vi "Interfaz grafica - corriente.vi"() -> ()   [LabVIEW 2024]
uses:
  160620 Optotune Lens Driver 4 Labview package/Hello Optotune Lens (30.06.2015)/Calibration.ctl
  <vilib>/DAQmx/read.llb/DAQmx Read (Analog 1D Wfm NChan NSamp).vi
  <vilib>/Analysis/2dsp.llb/Decimate (single shot, DBL).vi
  <vilib>/Utility/file.llb/Read Delimited Spreadsheet (string).vi
  <vilib>/Instr/_visa.llb/VISA Configure Serial Port (Instr).vi
  <vilib>/DAQmx/create/channels.llb/DAQmx Create Channel (AI-Voltage-Basic).vi
  <vilib>/DAQmx/configure/timing.llb/DAQmx Timing (Sample Clock).vi
  <vilib>/DAQmx/miscellaneous.llb/DAQmx Fill In Error Info.vi
  <vilib>/Waveform/WDTOps.llb/WDT Index Channel DBL.vi
  <vilib>/Analysis/2dsp.llb/Decimate (continuous, DBL).vi
  <vilib>/Utility/file.llb/Write Delimited Spreadsheet (string).vi
  <vilib>/Waveform/WDTOps.llb/WDT Get Waveform Time Array DBL.vi
  <vilib>/Analysis/NI_AALPro.lvlib
panel:
  out "Array 4":string[](array[string])
  out "Array 3":string[](array[string])
  out "Array 2":string[](array[string])
  out "Array":string[](array[string])
  out "Nombre 2":string
  in  "Restablecer Iniciales":bool
  in  "Incremento":dbl=0.1 format="%#_13g"
  out "Potencia derecho":dbl
  out "error out 4":errorcluster
  out "error out 3":errorcluster
  out "error out 2":errorcluster
  in  "Tab Control 3":enum32{"WL", "Video"}(tab)
  out "Waveform length":dbl[][](graph)
  in  "Minimo escala Y":dbl format="%#_13g"
  in  "Maximo escala Y":dbl format="%#_13g"
  in  "Escala autom. Y":u8=1
  in  "Escala autom. X":u8=1
  in  "Maximo escala X":dbl
  in  "Minimo escala X":dbl
  out "VISA resource name out":string
  in  "Tab Control 2":T1(tab)
  in  "DAQmx Physical Channel":tag
  in  "Frecuencia muestreo":i32=20000
  in  "tamaño buffer":i32=1000
  in  "factor decimacion":i32=20
  in  "Ganancia":u16(ring) items=["0.2"=51455, "1"=33023, "10"=49407, "20"=41215, "30"=57599, "40"=37119, "60"=53503, "80"=45311, "120"=61695, "157"=35071, ""=0]
  in  "Potencia inicial lente derecho":dbl(slide) scale=-3.0..3.0
  in  "Potencia inicial lente izquierdo":dbl(slide) scale=-3.0..3.0
  in  "VISA resource name":string="COM11"
  in  "VISA resource name 2":string="COM10"
  out "DPT INICIALES D":dbl
  out "DPT INICIALES I":dbl
  out "Potencia izquierdo":dbl
  in  "error in (no error) 5":errorcluster
  in  "error in (no error) 4":errorcluster
  in  "error in (no error) 3":errorcluster
  in  "error in (no error) 2":errorcluster
  in  "Calibration 4":T2={"Max Current A"=293.0, "Max Current B"=293.0, "UCL A"=300.0, "UCL B"=300.0, "LCL A"=0.0, "LCL B"=0.0} {"Max Current A" format="%#_g mA"; "Max Current B" format="%#_g mA"; "UCL A" format="%#_g mA"; "LCL A" format="%#_g mA"; "UCL B" format="%#_g mA"; "LCL B" format="%#_g mA"}
  out "ID 2":u16
  out "VISA resource name out 2":string
  out "Calibration 3":T2 {"Max Current A" format="%#_g mA"; "Max Current B" format="%#_g mA"; "UCL A" format="%#_g mA"; "LCL A" format="%#_g mA"; "UCL B" format="%#_g mA"; "LCL B" format="%#_g mA"}
  out "OK 2":bool
  out "Data 2":string
  out "Command to Port 2":string
  in  "Cola tipo 2":dbl[](array[numeric])
  out "Distancia":u32
  in  "Tamaño ventana WL":i32=60
  in  "Limite inferior WL":dbl=25.0 format="%#_13g"
  in  "Limite superior WL":dbl=50.0
  out "number":u32
  in  "Calibration":T2={"Max Current A"=293.0, "Max Current B"=293.0, "UCL A"=300.0, "UCL B"=300.0, "LCL A"=0.0, "LCL B"=0.0} {"Max Current A" format="%#_g mA"; "Max Current B" format="%#_g mA"; "UCL A" format="%#_g mA"; "LCL A" format="%#_g mA"; "UCL B" format="%#_g mA"; "LCL B" format="%#_g mA"}
  out "ID":u16
  out "Calibration 2":T2 {"Max Current A" format="%#_g mA"; "Max Current B" format="%#_g mA"; "UCL A" format="%#_g mA"; "LCL A" format="%#_g mA"; "UCL B" format="%#_g mA"; "LCL B" format="%#_g mA"}
  out "OK":bool
  out "Data":string
  out "Command to Port":string
  in  "DPT dif.":dbl
  out "error out":errorcluster
  in  "error in (no error)":errorcluster
  in  "WL":dbl
  in  "Cola tipo":dbl[](array[numeric])
  out "T button?":bool
  in  "Elegir menu Exp":bool
  in  "Elegir menu":bool
  out "path":path
  in  "Iniciar experimento":bool
  in  "Parar adquisicion":bool
  out "Enfermedad visual":string
  out "Edad":string
  out "Nombre":string
  out "Cedula":string
  in  "Carpeta":path=path "C:/Users/TGM1603/Documents/LabVIEW Data/Experimentos electrodos"
  in  "?":bool
  in  "Menu Principal":u16(ring) items=["Visualizacion general ", "Llevar a cabo un experimento", "Ajustar potencia inicial lentes"]
  in  "Menu experimentos":u16(ring) items=["Experimento 1", "Experimento 2", "Experimento 3", "Experimento 4"]
  in  "Tab Control":enum32{"Señal EMG", "Potencia y distancia"}(tab)
  out "Senal EMG":waveform(dbl)[](graph)
  in  "Escala automatica Y":u8
  in  "Escala automatica X":u8=1
  in  "X Scale.Range:Increment":dbl
  in  "X Scale.Range:Minimum":dbl
  in  "X Scale.Range:Maximum":dbl
  in  "Y Scale.Range:Minimum":dbl=-5.0
  in  "Y Scale.Range:Maximum":dbl=5.0
  in  "Escala Y min":dbl
  in  "Escala Y max":dbl
  in  "Auto scale Y":u8=1
  in  "Escala X max":dbl
  in  "Escala X min":dbl
  out "Potencia optica y distancia":dbl[][](graph)
  in  "Auto scale X":u8=1
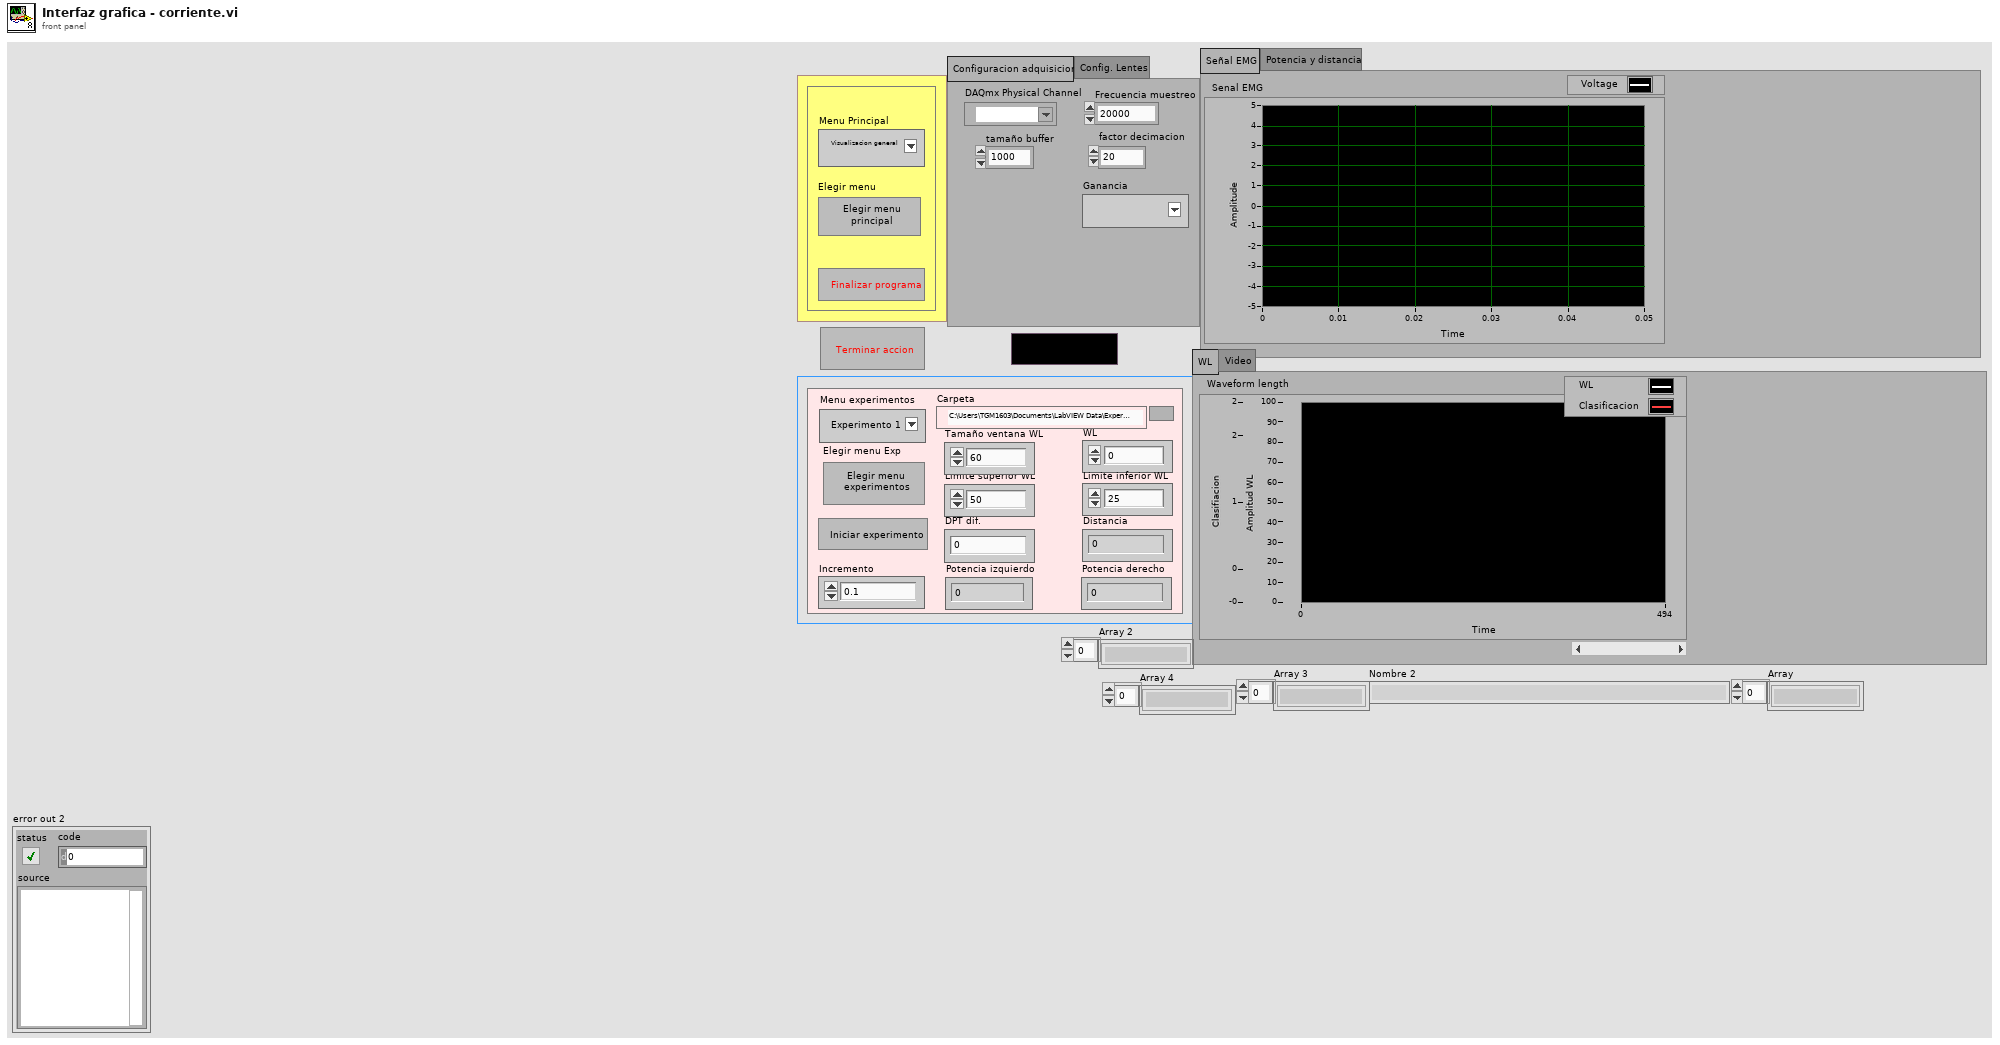
[diagram p1: front panel]
types:
  T1 = enum32{"Configuracion adquisicion", "Config. Lentes"}
  T2 = typedef "Calibration.ctl" = cluster{"Max Current A":dbl, "Max Current B":dbl, "UCL A":dbl, "UCL B":dbl, "LCL A":dbl, "LCL B":dbl}
  T3 = enum16{"Left Button", "Center Button", "Right Button", "Window Close"}
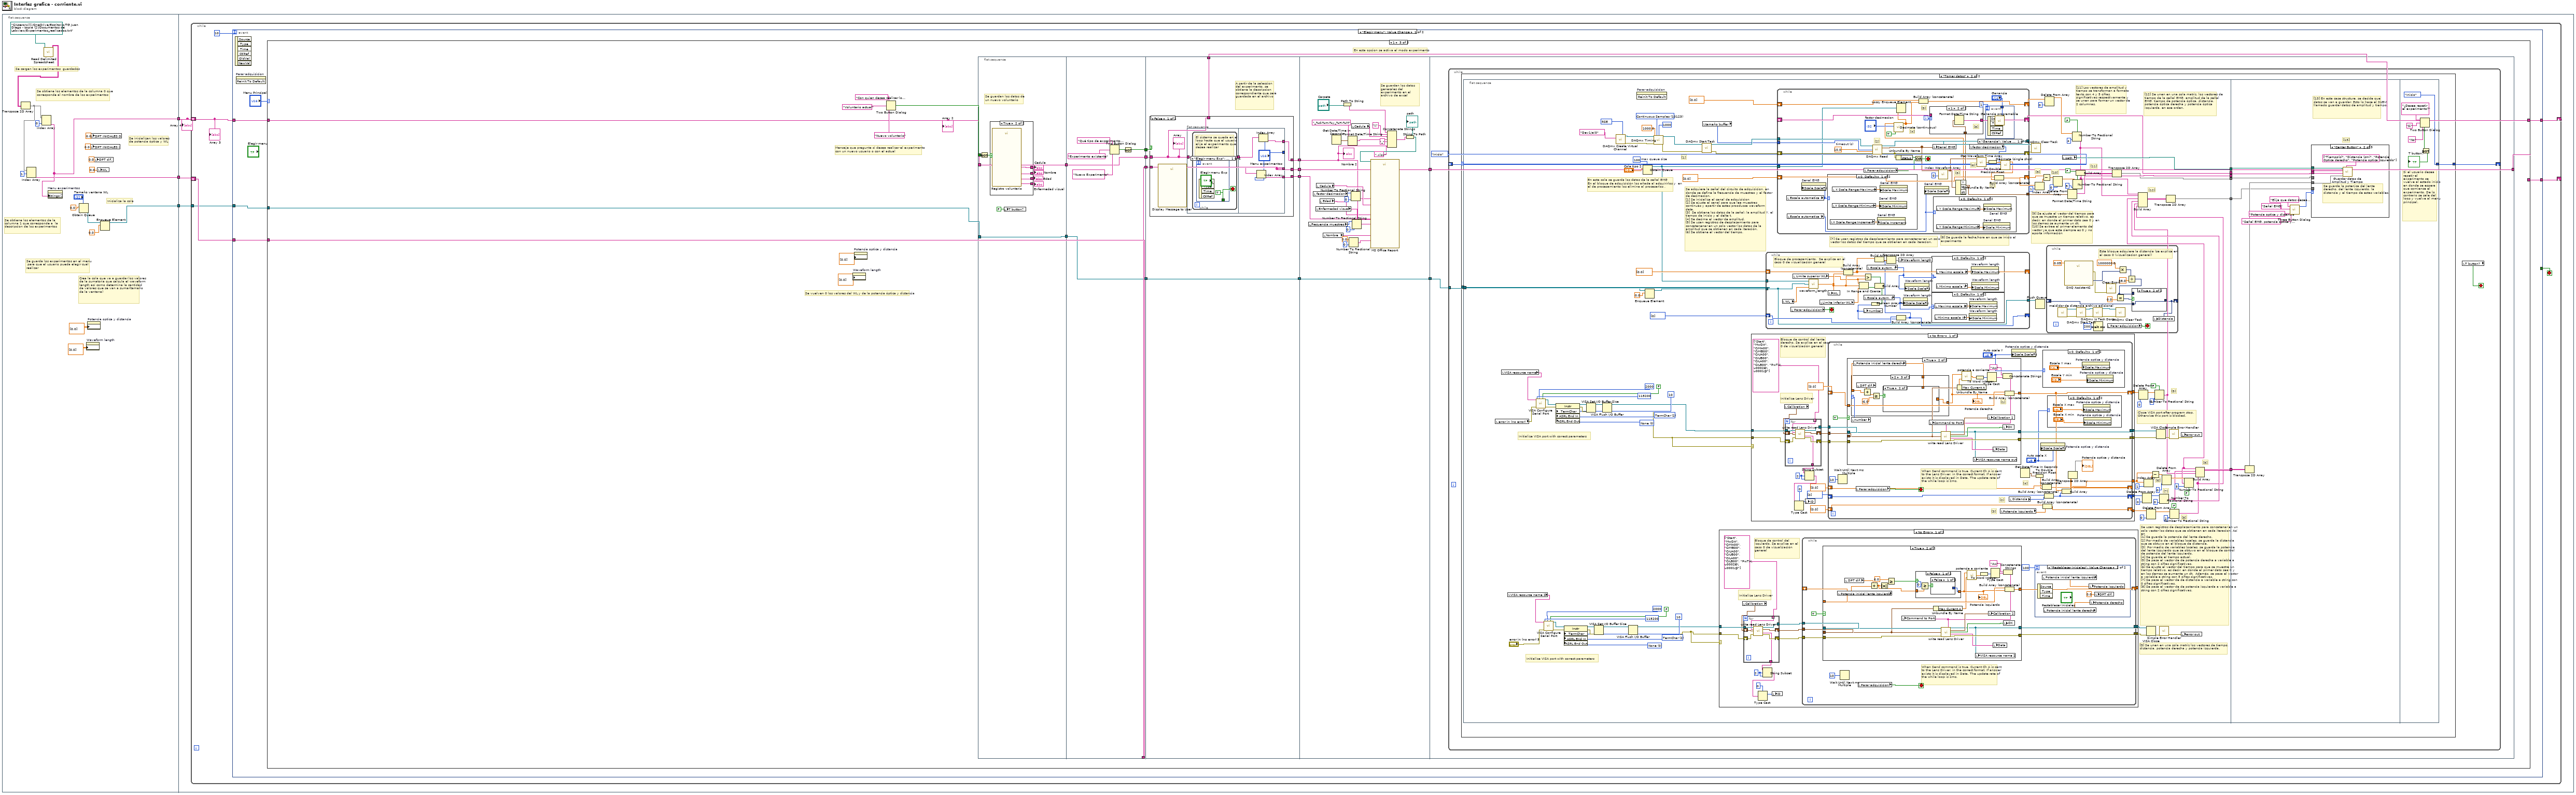
[diagram p0: block diagram]
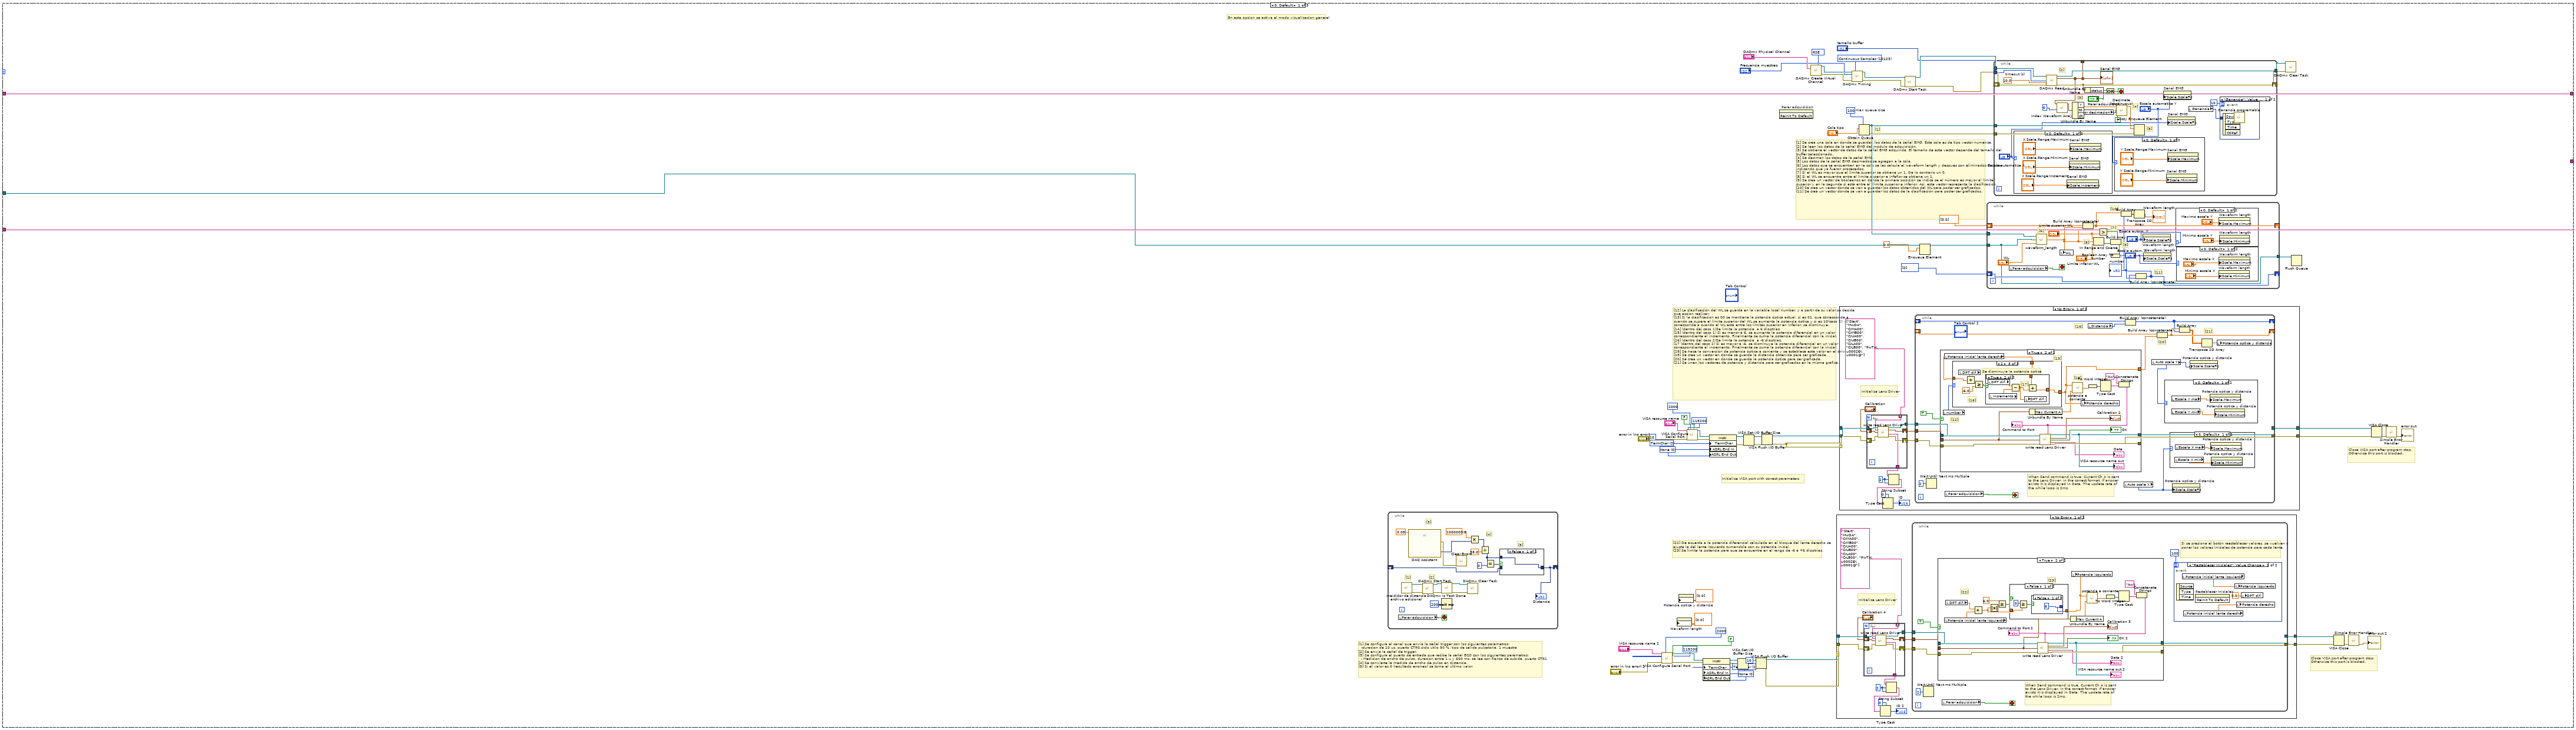
[diagram p2: hidden frame]
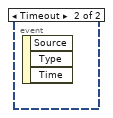
[diagram p3: hidden frame]
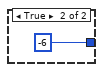
[diagram p5: hidden frame]
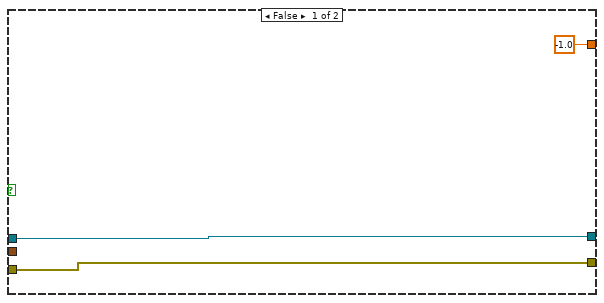
[diagram p11: hidden frame]
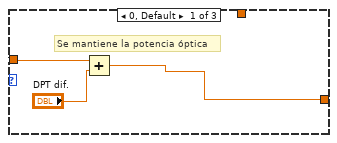
[diagram p12: hidden frame]
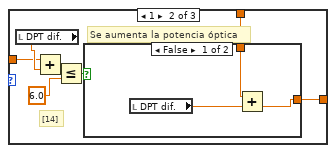
[diagram p13: hidden frame]
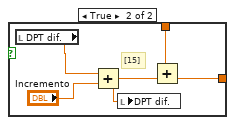
[diagram p14: hidden frame]
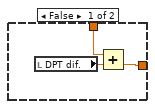
[diagram p15: hidden frame]
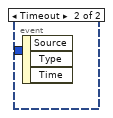
[diagram p19: hidden frame]
diagram:
  n1 = flat-sequence {
    tunnel: [w18] -> w3
    tunnel: [w15] -> w2
    tunnel: [w10] -> w1
    tunnel: w3 -> [w22]
    tunnel: w2 -> [w24]
    tunnel: w1 -> [w23]
    frame #0 {
      # "Se inicializan los valores\nde potencia óptica y WL"
      # "Inicializa la cola"
      # "Crea la cola que va a guardar los valores de la sumatoria que calcula el waveform length así como determina la cantidad de valores que se van a sumar(tamaño de la ventana)"
      # "Se obtiene los elementos de la columna 1 que corresponde a  la descripcion de los experimentos"
      # "Se obtiene los elementos de la columna 0 que corresponde al nombre de los experimentos"
      # "Se guarda los experimentos en el menu\n para que el usuario pueda elegir cual \nrealizar"
      # "Se cargan los experimentos  guardados"
      n2 = call-poly <vilib>:"Read Delimited Spreadsheet.vi"("file path (dialog if empty)"=path "C:/Users/willi/OneDrive/Escritorio/TG Juan Diego - copia (2)/Documentos de Labview/Experimentos_realizados.txt") -> ("all rows"=w19:string[][])  [unwired: 9 in, 5 out]
      n3 = Transpose 2D Array(2D array=w19) -> (transposed array=w16:string[][])
      n4 = Index Array(array=w16, index (row)=1) -> (element=w15:string[])  [unwired: 1 in]
      n5 = Index Array(array=w16, index (row)=0) -> (element=w18:string[])  [unwired: 1 in]
      n6 = property on="Menu experimentos" class="Ring (strict)"("Strings []"=w18) -> ()  [unwired: 2 in, 2 out]
      n7 = Obtain Queue(max queue size (-1, unlimited)="Tamaño ventana WL", element data type=0.0) -> (queue out=w13:refnum<queue>)  [unwired: 3 in, 2 out]
      n8 = property on="Waveform length" class="WFChart (strict)"("History Data"=dbl[][] [[0.0]]) -> ()  [unwired: 2 in, 2 out]
      n9 = property on="Potencia optica y distancia" class="WFChart (strict)"("History Data"=dbl[][] [[0.0]]) -> ()  [unwired: 2 in, 2 out]
      n10 = local write "DPT INICIALES D"(0.0 ("DPT INIT.1")) -> ()
      n11 = local write "DPT INICIALES I"(0.0 ("DPT INIT.2")) -> ()
      n12 = local write "DPT dif."(0.0 ("WL")) -> ()
      n13 = local write "WL"(0.0 ("WL")) -> ()
      n14 = Enqueue Element(queue=w13, element=0.0) -> (queue out=w10:refnum<queue>)  [unwired: 2 in, 2 out]
    }
    frame #1 {
      n15 = while {
        shift-right: [w30] -> _
        shift-left: w22 -> [w31]
        shift-right: [w28] -> _
        shift-left: w24 -> [w29]
        tunnel: w23 -> [w27]
        stop <- w26 stop-if-true
        n16 = event shown="[0] \"Elegir menu\": Value Change" {
          selector: _ -> [_ _]
          dyn-events: _ -> [_ _]
          timeout: 10 -> [_ _]
          tunnel: w31 -> [w37 w1042]
          tunnel: [w36 w1042] -> w30
          tunnel: w29 -> [w35 w1041]
          tunnel: [w34 w1041] -> w28
          tunnel: w27 -> [w32 _]
          tunnel: [_ "?"] -> w26
          event "Elegir menu": Value Change {
            n17 = event-data() -> ()  [unwired: 1 in, 6 out]
            n18 = invoke on="Parar adquisicion" class="Bool (strict)" method="Reinit To Default"() -> ()  [unwired: 3 in, 3 out]
            n19 = case shown="1" "Menu Principal" {
              tunnel: w37 -> [w104 w383 w503]
              tunnel: [w104 w383 w502] -> w36
              tunnel: w35 -> [w103 w382 w500]
              tunnel: [w103 w382 w499] -> w34
              tunnel: w32 -> [w93 _ w490]
              frame 0, Default {
                w38 = 10123 items=["Finite Samples"=10178, "Continuous Samples"=10123, "Hardware Timed Single Point"=12522] ("sample mode")
                w39 = 10083 items=["Default"=-1, "RSE"=10083, "NRSE"=10078, "Differential"=10106, "Pseudodifferential"=12529] ("input terminal configuration")
                w61 = u16 0 items=["None", "Last Bit", "TermChar", "Break"] ("Serial Settings:End Mode for Writes")
                w60 = u16 2 items=["None", "Last Bit", "TermChar"] ("Serial Settings:End Mode for Reads")
                w83 = u16 0 items=["None", "Last Bit", "TermChar", "Break"] ("Serial Settings:End Mode for Writes")
                w84 = u16 2 items=["None", "Last Bit", "TermChar"] ("Serial Settings:End Mode for Reads")
                w97 = 100  # max queue size
                # "[22] De acuerda a la potencia diferencial calculada en el bloque del lente derecho se ajusta la del lente izquierdo sumandola con su potencia inicial.\n[23] Se limita la potencia para que se encuentre en el rango de -6 a +6 dioptrías."
                # "[12] La clasificación del WL se guarda en la variable local number, y a partir de su valor se decide que accion realizar.\n[13] Si la clasificacion es 00 se mantiene la potencia óptica actual, si es 01, que corresponde a cuando se supera el limite superior del WL,se aumenta la potencia óptica y si es 10(caso 2), que corresponde a cuando el WL está entre los limites superior en inferior, se disminuye. \n[14] (dentro del caso 1)Se limita la potencia  a 6 dioptrías. \n[15] (dentro del caso 1) Si es menor a 6, se aumenta la potencia diferencial en un valor correspondiente al incremento. Finalmente se suma la potencia diferencial con la inicial.\n[16] (dentro del caso 2)Se limita la potencia  a -6 dioptrías.\n[17 (dentro del caso 2) Si es mayor a -6, se disminuye la potencia diferencial en un valor correspondiente al incremento. Finalmente se suma la potencia diferencial con la inicial.\n[18] Se hace la conversión de potencia óptica a corriente y se establece este valor en el driver.\n[19] Se crea un vector en donde se guarda la distancia obtenida para ser graficada.\n[20] Se crea un vector en donde se guarda la potencia óptica para ser graficada.\n[21] Se unen los vectores de potencia y distancia para ser graficados en la misma grafica."
                # "[1] Se crea una cola en donde se guardan los datos de la señal EMG. Esta cola es de tipo vector numerica.\n[2] Se leen los datos de la señal EMG del módulo de adquisición. \n[3] Se obtiene el vector de datos de la señal EMG adquirida. El tamaño de este vector depende del tamaño del buffer seleccionado.\n[4] Se deciman los datos de la señal EMG.\n[5] Los datos de la señal EMG decimados se agregan a la cola.\n[6] Los datos que se encuentran en la cola se les calcula el waveform length y después son eliminados de esta, indicando que ya fueron procesados. \n[7] Si el WL es mayor que el limite superior se obtiene un 1. De lo contrario un 0.\n[8] Si el WL se encuentra entre el límite superior e infefior se obtiene un 1.\n[9] Se crea un vector de booleanos en donde la primera posición se indica se el número es mayor al límite superior y en la segunda si está entre el  limite superior e inferior. Así, este vector representa la clasificación.\n[10] Se crea un vector donde se van a guardar los datos obtenidos del WL para poder ser graficados.\n[11] Se crea un vector donde se van a guardar los datos de la clasificación para poder ser graficados."
                # "[1]"
                # "En esta opcion se activa el modo visualizacion general"
                # "Close VISA port after program stop. Otherwise this port is blocked."
                # "[1] Se configura el canal que envía la señal trigger con los siguientes parametros:\n  -duracion de 10 us, puerto CTR0,ciclo utilo 50 %, tipo de salida pulsatoria, 1 muestra \n[2] Se envía la señal de trigger.\n[3] Se configura el puerto de entrada que recibe la señal ECO con los siguientes parámetros:\n  - Medicion de ancho de pulso, duracion entre 1 u y 600 ms, se lee con flanco de subida, puerto CTR1\n[4] Se convierte la medida de ancho de pulso en distancia.\n[5] Si el valor es 0 (resultado erroneo) se toma el último valor."
                # "Close VISA port after program stop. Otherwise this port is blocked."
                # "Initialize VISA port with correct parameters"
                n20 = while {
                  shift-right: [w172] -> _
                  shift-left: _ -> [w171]
                  stop <- w176 stop-if-true
                  # "[5]"
                  # "[4]"
                  # "[3]"
                  # "[2]"
                  # "[1]"
                  n21 = local read "Parar adquisicion"() -> (w176:bool)
                  n22 = call "meididor de distancia archivo adicional.vi"() -> ("error out"=w179:errorcluster, "task out"=w180:refnum<k21>)  [unwired: 10 in]
                  n23 = call "DAQ Assistant"("timeout (s)"=0.05) -> ("data"=w189:dynamicdata, "error out"=w177:errorcluster)  [unwired: 16 in, 1 out]
                  n24 = call <vilib>:"DAQmx Start Task.vi"("task/channels in"=w180, "error in"=w179) -> ("task out"=w183:refnum<k21>, "error out"=w184:errorcluster)  [unwired: 12 in]
                  n25 = call <vilib>:"DAQmx Is Task Done.vi"("task/channels in"=w183, "error in"=w184) -> ("task out"=w181:refnum<k21>, "error out"=w182:errorcluster)  [unwired: 11 in, 1 out]
                  n26 = Wait (ms)(milliseconds to wait=u32 200) -> ()  [unwired: 1 out]
                  n27 = call <vilib>:"Clear Errors.vi"("error in (no error)"=w177) -> ()  [unwired: 5 in, 2 out]
                  n28 = call <vilib>:"DAQmx Clear Task.vi"("task in"=w181, "error in"=w182) -> ()  [unwired: 13 in, 1 out]
                  n29 = Multiply(x=1000000.0, y=w189) -> (x*y=w187:dynamicdata)
                  n30 = Divide(x=w187, y=58.0) -> (x/y=w173:dynamicdata)
                  n31 = Equal?(x=w173, y=u16 0) -> (x = y?=w175:dynamicdata)
                  n32 = case shown="False" w175 {
                    tunnel: [w190 w191] -> w172
                    tunnel: w173 -> [w190 _]
                    tunnel: w171 -> [_ w191]
                    frame False {
                    }
                    frame True {
                    }
                  }
                  "Distancia" <- w172
                }
                n33 = call-poly "VISA Configure Serial Port"("VISA resource name"="VISA resource name 2", "timeout (10sec)"=u32 2000, "Enable Termination\nChar (T)"=FALSE ("Enable Termination\nChar (T)"), "baud rate (9600)"=u32 115200, "error in (no error)"="error in (no error) 2") -> ("VISA resource name out"=w56:refnum<visa-resource-name>, "error out"=w58:errorcluster)  [unwired: 9 in]
                n34 = property on="Waveform length" class="WFChart (strict)"("History Data"=dbl[][] [[0.0]]) -> ()  [unwired: 2 in, 2 out]
                n35 = property on="Potencia optica y distancia" class="WFChart (strict)"("History Data"=dbl[][] [[0.0]]) -> ()  [unwired: 2 in, 2 out]
                n36 = call-poly "VISA Configure Serial Port"("VISA resource name"="VISA resource name", "timeout (10sec)"=u32 2000, "Enable Termination\nChar (T)"=FALSE ("Enable Termination\nChar (T)"), "baud rate (9600)"=u32 115200, "error in (no error)"="error in (no error)") -> ("VISA resource name out"=w88:refnum<visa-resource-name>, "error out"=w86:errorcluster)  [unwired: 9 in]
                n37 = property class="Instr"(reference=w56, error in=w58, "TermChar"=u8 10 ("Message Based Settings:Termination Character"), "ASRL End In"=w60, "ASRL End Out"=w61) -> (reference out=w57:refnum<visa-resource-name>, error out=w59:errorcluster)
                n38 = property class="Instr"(reference=w88, error in=w86, "TermChar"=u8 10 ("Message Based Settings:Termination Character"), "ASRL End In"=w84, "ASRL End Out"=w83) -> (reference out=w87:refnum<visa-resource-name>, error out=w85:errorcluster)
                n39 = VISA Set I/O Buffer Size(VISA resource name=w57, error in (no error)=w59) -> (VISA resource name out=w64:refnum<visa-resource-name>, error out=w65:errorcluster)  [unwired: 2 in]
                n40 = VISA Set I/O Buffer Size(VISA resource name=w87, error in (no error)=w85) -> (VISA resource name out=w80:refnum<visa-resource-name>, error out=w79:errorcluster)  [unwired: 2 in]
                n41 = VISA Flush I/O Buffer(VISA resource name=w64, error in (no error)=w65) -> (VISA resource name out=w50:refnum<visa-resource-name>, error out=w51:errorcluster)  [unwired: 1 in]
                n42 = VISA Flush I/O Buffer(VISA resource name=w80, error in (no error)=w79) -> (VISA resource name out=w78:refnum<visa-resource-name>, error out=w73:errorcluster)  [unwired: 1 in]
                n43 = invoke on="Parar adquisicion" class="Bool (strict)" method="Reinit To Default"() -> ()  [unwired: 3 in, 3 out]
                n44 = call-poly <vilib>:"DAQmx Create Virtual Channel.vi"("input terminal configuration"=w39, "physical channels"="DAQmx Physical Channel") -> ("task out"=w45:refnum<k21>, "error out"=w44:errorcluster)  [unwired: 12 in]
                n45 = case shown="No Error" w51 {
                  tunnel: w51 -> [w118 w169]
                  tunnel: w50 -> [w117 w170]
                  tunnel: [w116 w169] -> w46
                  tunnel: [w115 w170] -> w47
                  frame No Error {
                    w113 = 2 ("length (rest)")
                    # "Initialize Lens Driver"
                    n46 = for {
                      tunnel: w117 -> [w167]
                      tunnel: [w164] -> w107
                      tunnel: string[] ["Start", "MwDA", "CrMA00", "CrMB00", "CrUA00", "CrUB00", "CrLA00", "CrLB00", "PwTA\u0002Ð\u0001@"] -> [w162] mode=indexing
                      tunnel: [w161] -> w106
                      shift-right: [w165] -> w108
                      shift-left: "Calibration 4" -> [w166]
                      shift-right: [w163] -> w109
                      shift-left: w118 -> [w168]
                      n47 = call "write read Lens Driver.vi"("VISA resource name"=w167, "command"=w162, "Calibration"=w166, "error in (no error)"=w168) -> ("VISA resource name out"=w164:refnum<visa-resource-name>, "Calibration 2"=w165:T2, "Data"=w161:string, "error out"=w163:errorcluster)  [unwired: 4 in, 4 out]
                    }
                    n48 = String Subset(string=w106, offset (0)=w113, length (rest)=w113) -> (substring=w111:string)
                    n49 = Type Cast(type=u16 0 ("length (rest)"), x=w111) -> (*(type *) &x=→"ID 2":u16)
                    n50 = while {
                      tunnel: [w121] -> w116
                      tunnel: [w122] -> w115
                      tunnel: w109 -> [w127]
                      tunnel: w108 -> [w126]
                      tunnel: w107 -> [w125]
                      stop <- w120 stop-if-true
                      # "Si se presiona el botón reestablecer valores, se vuelven a poner los valores iniciales de potencia para cada lente"
                      # "When Send command is true, Current Ch A is sent to the Lens Driver, in the correct format. If answer exists it is displayed in Data. The update rate of the while loop is 2ms."
                      n51 = Wait Until Next ms Multiple(millisecond multiple=u32 2) -> ()  [unwired: 1 out]
                      n52 = case shown="True" TRUE ("Send command") {
                        tunnel: [w132 w153] -> w121
                        tunnel: w127 -> [w132 w152]
                        tunnel: w126 -> [_ w134]
                        tunnel: w125 -> [w131 w151]
                        tunnel: [w131 w148] -> w122
                        frame False {
                        }
                        frame True {
                          # "[23]"
                          # "[22]"
                          n53 = local read "Potencia inicial lente izquierdo"() -> (w142:dbl)
                          n54 = local read "DPT dif."() -> (w143:dbl)
                          n55 = Add(x=w143, y=w142) -> (x+y=w138:dbl)
                          n56 = Absolute Value(x=w138) -> (abs(x)=w140:dbl)
                          n57 = Greater Or Equal?(x=6.0, y=w140) -> (x >= y?=w141:bool)
                          n58 = case shown="False" w141 {
                            tunnel: w138 -> [w156 w160]
                            tunnel: [w154 w160] -> w136
                            frame False {
                              n59 = Greater Or Equal?(x=u16 0, y=w156) -> (x >= y?=w157:bool)
                              n60 = case shown="False" w157 {
                                tunnel: [i16 6 ("x") i16 -6 ("x")] -> w154
                                frame False {
                                }
                                frame True {
                                }
                              }
                            }
                            frame True {
                            }
                          }
                          n61 = Unbundle By Name(w134) -> ("Max Current A"=w135:dbl)
                          n62 = local write "Potencia izquierdo"(w136) -> ()
                          n63 = call "potencia a corriente.vi"("Max current A"=w135, "Potencia"=w136) -> ("Corriente"=w137:dbl)
                          n64 = To Word Integer(number=w137) -> (16bit integer=w146:i16)
                          n65 = Type Cast(x=w146) -> (*(type *) &x=w145:string)  [unwired: 1 in]
                          n66 = Concatenate Strings("Aw", w145) -> (w144:string)
                          "Command to Port 2" <- w144
                          n67 = call "write read Lens Driver.vi"("VISA resource name"=w151, "command"=w144, "Calibration"=w134, "error in (no error)"=w152) -> ("VISA resource name out"=w148:refnum<visa-resource-name>, "Calibration 2"=→"Calibration 3":T2, "OK"=→"OK 2":bool, "Data"=→"Data 2":string, "error out"=w153:errorcluster)  [unwired: 4 in, 3 out]
                          "VISA resource name out 2" <- w148
                        }
                      }
                      n68 = local read "Parar adquisicion"() -> (w120:bool)
                      n69 = event shown="[0] \"Restablecer Iniciales\": Value Change" {
                        selector: _ -> [_ _]
                        dyn-events: _ -> [_ _]
                        timeout: 100 -> [_ _]
                        event "Restablecer Iniciales": Value Change {
                          n70 = event-data() -> ()  [unwired: 1 in, 3 out]
                          n71 = local read "Potencia inicial lente izquierdo"() -> (w128:dbl)
                          n72 = local read "Potencia inicial lente derecho"() -> (w129:dbl)
                          n73 = invoke on="Restablecer Iniciales" class="Bool" method="Reinit To Default"() -> ()  [unwired: 3 in, 3 out]
                          n74 = local write "Potencia izquierdo"(w128) -> ()
                          n75 = local write "Potencia derecho"(w129) -> ()
                          n76 = local write "DPT dif."(0.0 ("DPT dif.")) -> ()
                        }
                        event Timeout {
                          n77 = event-data() -> ()  [unwired: 1 in, 3 out]
                        }
                      }
                    }
                  }
                  frame Error {
                  }
                }
                n78 = case shown="No Error" w73 {
                  tunnel: w73 -> [w205 w289]
                  tunnel: w78 -> [w204 w290]
                  tunnel: [w203 w289] -> w76
                  tunnel: [w202 w290] -> w74
                  frame No Error {
                    w200 = 2 ("length (rest)")
                    # "Initialize Lens Driver"
                    n79 = for {
                      tunnel: w204 -> [w287]
                      tunnel: [w284] -> w194
                      tunnel: string[] ["Start", "MwDA", "CrMA00", "CrMB00", "CrUA00", "CrUB00", "CrLA00", "CrLB00", "PwTA\u0002Ð\u0001@"] -> [w282] mode=indexing
                      tunnel: [w281] -> w193
                      shift-right: [w285] -> w195
                      shift-left: "Calibration" -> [w286]
                      shift-right: [w283] -> w196
                      shift-left: w205 -> [w288]
                      n80 = call "write read Lens Driver.vi"("VISA resource name"=w287, "command"=w282, "Calibration"=w286, "error in (no error)"=w288) -> ("VISA resource name out"=w284:refnum<visa-resource-name>, "Calibration 2"=w285:T2, "Data"=w281:string, "error out"=w283:errorcluster)  [unwired: 4 in, 4 out]
                    }
                    n81 = String Subset(string=w193, offset (0)=w200, length (rest)=w200) -> (substring=w198:string)
                    n82 = Type Cast(type=u16 0 ("length (rest)"), x=w198) -> (*(type *) &x=→"ID":u16)
                    n83 = while {
                      tunnel: [w217] -> w203
                      tunnel: [w218] -> w202
                      tunnel: w196 -> [w223]
                      tunnel: w195 -> [w222]
                      tunnel: w194 -> [w221]
                      shift-right: [w208] -> _
                      shift-left: _ -> [w212]
                      shift-right: [w209] -> _
                      shift-left: _ -> [w211]
                      stop <- w216 stop-if-true
                      # "[21]"
                      # "[20]"
                      # "[19]"
                      # "When Send command is true, Current Ch A is sent to the Lens Driver, in the correct format. If answer exists it is displayed in Data. The update rate of the while loop is 2ms."
                      n84 = Wait Until Next ms Multiple(millisecond multiple=u32 2) -> ()  [unwired: 1 out]
                      n85 = case shown="True" TRUE ("Send command") {
                        tunnel: [w230 w247] -> w217
                        tunnel: w223 -> [w230 w246]
                        tunnel: w222 -> [_ w233]
                        tunnel: w221 -> [w229 w245]
                        tunnel: [w229 w242] -> w218
                        tunnel: [-1.0 ("DPT") w235] -> w210
                        frame False {
                        }
                        frame True {
                          # "[18]"
                          # "[13]"
                          # "[12]"
                          n86 = local read "number"() -> (w237:u32)
                          n87 = local read "Potencia inicial lente derecho"() -> (w236:dbl)
                          n88 = case shown="2" w237 {
                            tunnel: [w249 w257 w272] -> w235
                            tunnel: w236 -> [w250 w252 w267]
                            tunnel: w236 -> [_ w251 w266]
                            frame 0, Default {
                              # "Se mantiene la potencia óptica"
                              n89 = Add(x=w250, y="DPT dif.") -> (x+y=w249:dbl)
                            }
                            frame 1 {
                              # "[14]"
                              # "Se aumenta la potencia óptica"
                              n90 = local read "DPT dif."() -> (w253:dbl)
                              n91 = Add(x=w252, y=w253) -> (x+y=w254:dbl)
                              n92 = Less Or Equal?(x=w254, y=6.0) -> (x <= y?=w256:bool)
                              n93 = case shown="False" w256 {
                                tunnel: [w259 w262] -> w257
                                tunnel: w251 -> [w258 w261]
                                frame False {
                                n94 = local read "DPT dif."() -> (w260:dbl)
                                n95 = Add(x=w258, y=w260) -> (x+y=w259:dbl)
                                }
                                frame True {
                                # "[15]"
                                n96 = local read "DPT dif."() -> (w263:dbl)
                                n97 = Add(x=w263, y="Incremento") -> (x+y=w264:dbl)
                                n98 = local write "DPT dif."(w264) -> ()
                                n99 = Add(x=w261, y=w264) -> (x+y=w262:dbl)
                                }
                              }
                            }
                            frame 2 {
                              # "[16]"
                              # "Se disminuye la potencia óptica"
                              n100 = local read "DPT dif."() -> (w271:dbl)
                              n101 = Add(x=w271, y=w267) -> (x+y=w268:dbl)
                              n102 = Greater Or Equal?(x=w268, y=-6.0) -> (x >= y?=w269:bool)
                              n103 = case shown="True" w269 {
                                tunnel: [w274 w278] -> w272
                                tunnel: w266 -> [w273 w277]
                                frame False {
                                n104 = local read "DPT dif."() -> (w275:dbl)
                                n105 = Add(x=w273, y=w275) -> (x+y=w274:dbl)
                                }
                                frame True {
                                # "[17]"
                                n106 = local read "DPT dif."() -> (w280:dbl)
                                n107 = local read "Incremento"() -> (w276:dbl)
                                n108 = Subtract(x=w280, y=w276) -> (x-y=w279:dbl)
                                n109 = local write "DPT dif."(w279) -> ()
                                n110 = Add(x=w277, y=w279) -> (x+y=w278:dbl)
                                }
                              }
                            }
                          }
                          n111 = Unbundle By Name(w233) -> ("Max Current A"=w232:dbl)
                          n112 = call "potencia a corriente.vi"("Max current A"=w232, "Potencia"=w235) -> ("Corriente"=w234:dbl)
                          n113 = local write "Potencia derecho"(w235) -> ()
                          n114 = To Word Integer(number=w234) -> (16bit integer=w240:i16)
                          n115 = Type Cast(x=w240) -> (*(type *) &x=w239:string)  [unwired: 1 in]
                          n116 = Concatenate Strings("Aw", w239) -> (w238:string)
                          "Command to Port" <- w238
                          n117 = call "write read Lens Driver.vi"("VISA resource name"=w245, "command"=w238, "Calibration"=w233, "error in (no error)"=w246) -> ("VISA resource name out"=w242:refnum<visa-resource-name>, "Calibration 2"=→"Calibration 2":T2, "OK"=→"OK":bool, "Data"=→"Data":string, "error out"=w247:errorcluster)  [unwired: 4 in, 3 out]
                          "VISA resource name out" <- w242
                        }
                      }
                      n118 = local read "Parar adquisicion"() -> (w216:bool)
                      n119 = local read "Distancia"() -> (w213:u32)
                      n120 = local read "Auto scale X"() -> (w214:u8)
                      n121 = Build Array (concatenate)(w212, w213) -> (w208:u32[])
                      n122 = local read "Auto scale Y"() -> (w215:u8)
                      n123 = Build Array (concatenate)(w211, w210) -> (w209:dbl[])
                      n124 = case shown="0, Default" w215 {
                        frame 0, Default {
                          n125 = local read "Escala Y max"() -> (w227:dbl)
                          n126 = local read "Escala Y min"() -> (w226:dbl)
                          n127 = property on="Potencia optica y distancia" class="WFChart (strict)"("YScale.Maximum"=w227) -> ()  [unwired: 2 in, 2 out]
                          n128 = property on="Potencia optica y distancia" class="WFChart (strict)"("YScale.Minimum"=w226) -> ()  [unwired: 2 in, 2 out]
                        }
                        frame 1 {
                        }
                      }
                      n129 = case shown="0, Default" w214 {
                        frame 0, Default {
                          n130 = local read "Escala X min"() -> (w224:dbl)
                          n131 = local read "Escala X max"() -> (w225:dbl)
                          n132 = property on="Potencia optica y distancia" class="WFChart (strict)"("XScale.Maximum"=w225) -> ()  [unwired: 2 in, 2 out]
                          n133 = property on="Potencia optica y distancia" class="WFChart (strict)"("XScale.Minimum"=w224) -> ()  [unwired: 2 in, 2 out]
                        }
                        frame 1 {
                        }
                      }
                      n134 = property on="Potencia optica y distancia" class="WFChart (strict)"("XScale.ScaleFit"=w214) -> ()  [unwired: 2 in, 2 out]
                      n135 = Build Array(w209, w208) -> (w207:dbl[][])
                      n136 = property on="Potencia optica y distancia" class="WFChart (strict)"("YScale.ScaleFit"=w215) -> ()  [unwired: 2 in, 2 out]
                      n137 = Transpose 2D Array(2D array=w207) -> (transposed array=w206:dbl[][])
                      n138 = local write "Potencia optica y distancia"(w206) -> ()
                    }
                  }
                  frame Error {
                  }
                }
                n139 = call-poly <vilib>:"DAQmx Timing.vi"("task/channels in"=w45, "sample mode"=w38, "rate"="Frecuencia muestreo", "error in"=w44) -> ("task out"=w43:refnum<k21>, "error out"=w42:errorcluster)  [unwired: 10 in]
                n140 = Obtain Queue(max queue size (-1, unlimited)=w97, element data type="Cola tipo") -> (queue out=w94:refnum<queue>, error out=w95:errorcluster)  [unwired: 3 in, 1 out]
                n141 = call <vilib>:"DAQmx Start Task.vi"("task/channels in"=w43, "error in"=w42) -> ("task out"=w102:refnum<k21>, "error out"=w101:errorcluster)  [unwired: 12 in]
                n142 = Enqueue Element(queue=w93, element=0.0) -> (queue out=w70:refnum<queue>)  [unwired: 2 in, 2 out]
                n143 = while {
                  tunnel: w70 -> [w292]
                  tunnel: w94 -> [w309]
                  shift-right: [w295] -> _
                  shift-left: dbl[] [0.0] -> [w306]
                  shift-right: [w294] -> _
                  shift-left: u32[] [0] -> [w296]
                  tunnel: [w292] -> w68
                  stop <- w307 stop-if-true
                  # "[11]"
                  # "[10]"
                  # "[9]"
                  # "[8]"
                  # "[7]"
                  # "[6]"
                  n144 = local read "Parar adquisicion"() -> (w307:bool)
                  n145 = call "waveform_length.vi"("WL"="WL", "Cola WL"=w292, "Datos entrada"=w309) -> ("WL 2"=w304:dbl)
                  n146 = local write "WL"(w304) -> ()
                  n147 = Build Array (concatenate)(w306, w304) -> (w295:dbl[])
                  n148 = In Range and Coerce(upper limit="Limite superior WL", x=w304, lower limit="Limite inferior WL") -> (In Range?=w302:bool)  [unwired: 1 out]
                  n149 = Greater?(x=w304, y="Limite superior WL") -> (0:w303:bool)
                  n150 = Build Array(w303, w302) -> (w301:bool[])
                  n151 = Boolean Array To Number(Boolean array=w301) -> (number=w297:u32)
                  "number" <- w297
                  n152 = Build Array (concatenate)(w296, w297) -> (w294:u32[])
                  n153 = Build Array(w295, w294) -> (w293:dbl[][])
                  n154 = Transpose 2D Array(2D array=w293) -> (transposed array=→"Waveform length":dbl[][])
                  n155 = property on="Waveform length" class="WFChart (strict)"("YScale.ScaleFit"="Escala autom. Y") -> ()  [unwired: 2 in, 2 out]
                  n156 = property on="Waveform length" class="WFChart (strict)"("XScale.ScaleFit"="Escala autom. X") -> ()  [unwired: 2 in, 2 out]
                  n157 = case shown="0, Default" "Escala autom. Y" {
                    frame 0, Default {
                      n158 = property on="Waveform length" class="WFChart (strict)"("YScale.Maximum"="Maximo escala Y") -> ()  [unwired: 2 in, 2 out]
                      n159 = property on="Waveform length" class="WFChart (strict)"("YScale.Minimum"="Minimo escala Y") -> ()  [unwired: 2 in, 2 out]
                    }
                    frame 1 {
                    }
                  }
                  n160 = case shown="0, Default" "Escala autom. X" {
                    frame 0, Default {
                      n161 = property on="Waveform length" class="WFChart (strict)"("XScale.Minimum"="Minimo escala X") -> ()  [unwired: 2 in, 2 out]
                      n162 = property on="Waveform length" class="WFChart (strict)"("XScale.Maximum"="Maximo escala X") -> ()  [unwired: 2 in, 2 out]
                    }
                    frame 1 {
                    }
                  }
                }
                n163 = while {
                  tunnel: w102 -> [w335]
                  tunnel: "tamaño buffer" -> [w332]
                  tunnel: [w333] -> w98
                  shift-right: [w330] -> w99
                  shift-left: w101 -> [w334]
                  tunnel: [w324] -> _
                  tunnel: w94 -> [w320]
                  tunnel: w95 -> [w319]
                  stop <- w329 stop-if-true
                  w328 = 10.0  # timeout (s)
                  # "[5]"
                  # "[4]"
                  # "[3]"
                  # "[2]"
                  n164 = case shown="0, Default" "Escala automatica X" {
                    frame 0, Default {
                      n165 = property on="Senal EMG" class="WFGraph (strict)"("XScale.Increment"="X Scale.Range:Increment") -> ()  [unwired: 2 in, 2 out]
                      n166 = property on="Senal EMG" class="WFGraph (strict)"("XScale.Minimum"="X Scale.Range:Minimum") -> ()  [unwired: 2 in, 2 out]
                      n167 = property on="Senal EMG" class="WFGraph (strict)"("XScale.Maximum"="X Scale.Range:Maximum") -> ()  [unwired: 2 in, 2 out]
                    }
                    frame 1 {
                    }
                  }
                  n168 = call-poly <vilib>:"DAQmx Read.vi"("task/channels in"=w335, "number of samples per channel"=w332, "timeout"=w328, "error in"=w334) -> ("task out"=w333:refnum<k21>, "data"=w324:waveform(dbl)[], "error out"=w330:errorcluster)  [unwired: 9 in]
                  "Senal EMG" <- w324
                  n169 = call-poly <vilib>:"Index Waveform Array.vi"("index"=0, "waveform array"=w324) -> ("waveform"=w325:waveform(dbl))  [unwired: 8 in, 1 out]
                  n170 = Unbundle By Name(w325) -> ("Y"=w322:dbl[])  [unwired: 2 out]
                  n171 = local read "factor decimacion"() -> (w321:i32)
                  n172 = Unbundle By Name(w330) -> ("status"=w331:bool)
                  n173 = Or(x=w331, y="Parar adquisicion") -> (x .or. y?=w329:bool)
                  n174 = case shown="0, Default" "Escala automatica Y" {
                    frame 0, Default {
                      n175 = property on="Senal EMG" class="WFGraph (strict)"("YScale.Minimum"="Y Scale.Range:Minimum") -> ()  [unwired: 2 in, 2 out]
                      n176 = property on="Senal EMG" class="WFGraph (strict)"("YScale.Maximum"="Y Scale.Range:Maximum") -> ()  [unwired: 2 in, 2 out]
                    }
                    frame 1 {
                    }
                  }
                  n177 = call-poly <vilib>:"Decimate (continuous).vi"("averaging"=TRUE, "decimating factor"=w321, "X"=w322) -> ("Decimated Array"=w318:dbl[])  [unwired: 7 in, 1 out]
                  n178 = Lossy Enqueue Element(queue=w320, element=w318, error in (no error)=w319) -> ()  [unwired: 4 out]
                  n179 = property on="Senal EMG" class="WFGraph (strict)"("YScale.ScaleFit"="Escala automatica Y") -> ()  [unwired: 2 in, 2 out]
                  n180 = property on="Senal EMG" class="WFGraph (strict)"("XScale.ScaleFit"="Escala automatica X") -> ()  [unwired: 2 in, 2 out]
                  n181 = local read "Ganancia"() -> (w315:u16)
                  n182 = event shown="[0] \"Ganancia\": Value Change" {
                    selector: _ -> [_ _]
                    dyn-events: _ -> [_ _]
                    timeout: 10 -> [_ _]
                    tunnel: w315 -> [w336 _]
                    event "Ganancia": Value Change {
                      n183 = event-data() -> ()  [unwired: 1 in, 4 out]
                      n184 = call "Ganancia programable.vi"("MOSI data"=w336) -> ()
                    }
                    event Timeout {
                      n185 = event-data() -> ()  [unwired: 1 in, 3 out]
                    }
                  }
                }
                n186 = call <vilib>:"DAQmx Clear Task.vi"("task in"=w98, "error in"=w99) -> ()  [unwired: 13 in, 1 out]
                n187 = Flush Queue(queue=w68) -> ()  [unwired: 1 in, 3 out]
                n188 = VISA Close(VISA resource name=w47, error in (no error)=w46) -> (error out=w48:errorcluster)
                n189 = call <vilib>:"Simple Error Handler.vi"("error in (no error)"=w48) -> ("error out"=→"error out 2":errorcluster)  [unwired: 4 in, 4 out]
                n190 = VISA Close(VISA resource name=w74, error in (no error)=w76) -> (error out=w77:errorcluster)
                n191 = call <vilib>:"Simple Error Handler.vi"("error in (no error)"=w77) -> ("error out"=→"error out":errorcluster)  [unwired: 4 in, 4 out]
              }
              frame 2 {
                w362 = u16 0 items=["None", "Last Bit", "TermChar", "Break"] ("Serial Settings:End Mode for Writes")
                w361 = u16 2 items=["None", "Last Bit", "TermChar"] ("Serial Settings:End Mode for Reads")
                w375 = u16 0 items=["None", "Last Bit", "TermChar", "Break"] ("Serial Settings:End Mode for Writes")
                w374 = u16 2 items=["None", "Last Bit", "TermChar"] ("Serial Settings:End Mode for Reads")
                # "En esta opcion se configura la potencia inicial de los lentes"
                # "Close VISA port after program stop. Otherwise this port is blocked."
                # "Close VISA port after program stop. Otherwise this port is blocked."
                # "PwTA command to set temperature limits: PwTA as ASCII characters followed by 45 and 20 degrees in binary code."
                # "Initialize VISA port with correct parameters"
                # "PwTA command to set temperature limits: PwTA as ASCII characters followed by 45 and 20 degrees in binary code."
                # "Initialize VISA port with correct parameters"
                n192 = local read "VISA resource name"() -> (w352:string)
                n193 = call-poly "VISA Configure Serial Port"("VISA resource name"=w352, "timeout (10sec)"=u32 2000, "Enable Termination\nChar (T)"=FALSE ("Enable Termination\nChar (T)"), "baud rate (9600)"=u32 115200, "error in (no error)"="error in (no error) 3") -> ("VISA resource name out"=w357:refnum<visa-resource-name>, "error out"=w359:errorcluster)  [unwired: 9 in]
                n194 = property class="Instr"(reference=w357, error in=w359, "TermChar"=u8 10 ("Message Based Settings:Termination Character"), "ASRL End In"=w361, "ASRL End Out"=w362) -> (reference out=w358:refnum<visa-resource-name>, error out=w360:errorcluster)
                n195 = VISA Set I/O Buffer Size(VISA resource name=w358, error in (no error)=w360) -> (VISA resource name out=w364:refnum<visa-resource-name>, error out=w365:errorcluster)  [unwired: 2 in]
                n196 = VISA Flush I/O Buffer(VISA resource name=w364, error in (no error)=w365) -> (VISA resource name out=w351:refnum<visa-resource-name>, error out=w350:errorcluster)  [unwired: 1 in]
                n197 = case shown="No Error" w350 {
                  tunnel: w350 -> [w397 w431]
                  tunnel: w351 -> [w396 w432]
                  tunnel: [w395 w431] -> w346
                  tunnel: [w394 w432] -> w347
                  frame No Error {
                    w393 = 2 ("length (rest)")
                    # "Initialize Lens Driver"
                    n198 = local read "Calibration"() -> (w385:T2)
                    n199 = for {
                      tunnel: w396 -> [w429]
                      tunnel: [w426] -> w388
                      tunnel: string[] ["Start", "MwDA", "CrMA00", "CrMB00", "CrUA00", "CrUB00", "CrLA00", "CrLB00", "PwTA\u0002Ð\u0001@"] -> [w424] mode=indexing
                      tunnel: [w423] -> w387
                      shift-right: [w427] -> w389
                      shift-left: w385 -> [w428]
                      shift-right: [w425] -> w390
                      shift-left: w397 -> [w430]
                      n200 = call "write read Lens Driver.vi"("VISA resource name"=w429, "command"=w424, "Calibration"=w428, "error in (no error)"=w430) -> ("VISA resource name out"=w426:refnum<visa-resource-name>, "Calibration 2"=w427:T2, "Data"=w423:string, "error out"=w425:errorcluster)  [unwired: 4 in, 4 out]
                    }
                    n201 = String Subset(string=w387, offset (0)=w393, length (rest)=w393) -> (substring=w391:string)
                    n202 = Type Cast(type=u16 0 ("length (rest)"), x=w391) -> (*(type *) &x=w386:u16)
                    n203 = local write "ID"(w386) -> ()
                    n204 = while {
                      tunnel: [w399] -> w395
                      tunnel: [w400] -> w394
                      tunnel: w390 -> [w405]
                      tunnel: w389 -> [w404]
                      tunnel: w388 -> [w403]
                      stop <- w398 stop-if-true
                      # "When Send command is true, Current Ch A is sent to the Lens Driver, in the correct format. If answer exists it is displayed in Data. The update rate of the while loop is 2ms."
                      n205 = Wait Until Next ms Multiple(millisecond multiple=u32 2) -> ()  [unwired: 1 out]
                      n206 = case shown="True" TRUE ("Send command") {
                        tunnel: [w407 w422] -> w399
                        tunnel: w405 -> [w407 w421]
                        tunnel: w404 -> [_ w412]
                        tunnel: w403 -> [w406 w420]
                        tunnel: [w406 w413] -> w400
                        frame False {
                        }
                        frame True {
                          n207 = Unbundle By Name(w412) -> ("Max Current A"=w411:dbl)
                          n208 = call "potencia a corriente.vi"("Max current A"=w411, "Potencia"="Potencia inicial lente derecho") -> ("Corriente"=w409:dbl)
                          n209 = To Word Integer(number=w409) -> (16bit integer=w419:i16)
                          n210 = Type Cast(x=w419) -> (*(type *) &x=w418:string)  [unwired: 1 in]
                          n211 = Concatenate Strings("Aw", w418) -> (w415:string)
                          n212 = local write "Command to Port"(w415) -> ()
                          n213 = call "write read Lens Driver.vi"("VISA resource name"=w420, "command"=w415, "Calibration"=w412, "error in (no error)"=w421) -> ("VISA resource name out"=w413:refnum<visa-resource-name>, "Calibration 2"=w417:T2, "OK"=w416:bool, "Data"=w414:string, "error out"=w422:errorcluster)  [unwired: 4 in, 3 out]
                          n214 = local write "VISA resource name out"(w413) -> ()
                          n215 = local write "Calibration 2"(w417) -> ()
                          n216 = local write "Data"(w414) -> ()
                          n217 = local write "OK"(w416) -> ()
                          "DPT INICIALES D" <- "Potencia inicial lente derecho"
                        }
                      }
                      n218 = local read "Parar adquisicion"() -> (w398:bool)
                    }
                  }
                  frame Error {
                  }
                }
                n219 = VISA Close(VISA resource name=w347, error in (no error)=w346) -> (error out=w349:errorcluster)
                n220 = call <vilib>:"Simple Error Handler.vi"("error in (no error)"=w349) -> ("error out"=→"error out 3":errorcluster)  [unwired: 4 in, 4 out]
                n221 = local read "VISA resource name 2"() -> (w366:string)
                n222 = call-poly "VISA Configure Serial Port"("VISA resource name"=w366, "timeout (10sec)"=u32 2000, "Enable Termination\nChar (T)"=FALSE ("Enable Termination\nChar (T)"), "baud rate (9600)"=u32 115200, "error in (no error)"="error in (no error) 4") -> ("VISA resource name out"=w370:refnum<visa-resource-name>, "error out"=w372:errorcluster)  [unwired: 9 in]
                n223 = property class="Instr"(reference=w370, error in=w372, "TermChar"=u8 10 ("Message Based Settings:Termination Character"), "ASRL End In"=w374, "ASRL End Out"=w375) -> (reference out=w371:refnum<visa-resource-name>, error out=w373:errorcluster)
                n224 = VISA Set I/O Buffer Size(VISA resource name=w371, error in (no error)=w373) -> (VISA resource name out=w377:refnum<visa-resource-name>, error out=w378:errorcluster)  [unwired: 2 in]
                n225 = VISA Flush I/O Buffer(VISA resource name=w377, error in (no error)=w378) -> (VISA resource name out=w380:refnum<visa-resource-name>, error out=w379:errorcluster)  [unwired: 1 in]
                n226 = case shown="No Error" w379 {
                  tunnel: w379 -> [w446 w486]
                  tunnel: w380 -> [w445 w487]
                  tunnel: [w444 w486] -> w343
                  tunnel: [w443 w487] -> w342
                  frame No Error {
                    w442 = 2 ("length (rest)")
                    # "Initialize Lens Driver"
                    n227 = local read "Calibration"() -> (w434:T2)
                    n228 = for {
                      tunnel: w445 -> [w484]
                      tunnel: [w481] -> w437
                      tunnel: string[] ["Start", "MwDA", "CrMA00", "CrMB00", "CrUA00", "CrUB00", "CrLA00", "CrLB00", "PwTA\u0002Ð\u0001@"] -> [w479] mode=indexing
                      tunnel: [w478] -> w436
                      shift-right: [w482] -> w438
                      shift-left: w434 -> [w483]
                      shift-right: [w480] -> w439
                      shift-left: w446 -> [w485]
                      n229 = call "write read Lens Driver.vi"("VISA resource name"=w484, "command"=w479, "Calibration"=w483, "error in (no error)"=w485) -> ("VISA resource name out"=w481:refnum<visa-resource-name>, "Calibration 2"=w482:T2, "Data"=w478:string, "error out"=w480:errorcluster)  [unwired: 4 in, 4 out]
                    }
                    n230 = String Subset(string=w436, offset (0)=w442, length (rest)=w442) -> (substring=w440:string)
                    n231 = Type Cast(type=u16 0 ("length (rest)"), x=w440) -> (*(type *) &x=w435:u16)
                    n232 = local write "ID"(w435) -> ()
                    n233 = while {
                      tunnel: [w448] -> w444
                      tunnel: [w449] -> w443
                      tunnel: w439 -> [w454]
                      tunnel: w438 -> [w453]
                      tunnel: w437 -> [w452]
                      stop <- w447 stop-if-true
                      # "When Send command is true, Current Ch A is sent to the Lens Driver, in the correct format. If answer exists it is displayed in Data. The update rate of the while loop is 2ms."
                      n234 = Wait Until Next ms Multiple(millisecond multiple=u32 2) -> ()  [unwired: 1 out]
                      n235 = case shown="True" TRUE ("Send command") {
                        tunnel: [w456 w477] -> w448
                        tunnel: w454 -> [w456 w476]
                        tunnel: w453 -> [_ w464]
                        tunnel: w452 -> [w455 w475]
                        tunnel: [w455 w465] -> w449
                        frame False {
                        }
                        frame True {
                          n236 = Unbundle By Name(w464) -> ("Max Current A"=w463:dbl)
                          n237 = Multiply(x=15.8, y="Potencia inicial lente izquierdo") -> (x*y=w461:dbl)
                          n238 = Add(x=-6.8, y=w461) -> (x+y=w459:dbl)
                          n239 = Divide(x=w459, y=w463) -> (x/y=w462:dbl)
                          n240 = Multiply(x=4096.0, y=w462) -> (x*y=w473:dbl)
                          n241 = To Word Integer(number=w473) -> (16bit integer=w472:i16)
                          n242 = Type Cast(x=w472) -> (*(type *) &x=w471:string)  [unwired: 1 in]
                          n243 = Concatenate Strings("Aw", w471) -> (w467:string)
                          n244 = local write "Command to Port"(w467) -> ()
                          n245 = call "write read Lens Driver.vi"("VISA resource name"=w475, "command"=w467, "Calibration"=w464, "error in (no error)"=w476) -> ("VISA resource name out"=w465:refnum<visa-resource-name>, "Calibration 2"=w469:T2, "OK"=w468:bool, "Data"=w466:string, "error out"=w477:errorcluster)  [unwired: 4 in, 3 out]
                          n246 = local write "VISA resource name out 2"(w465) -> ()
                          n247 = local write "Calibration 2"(w469) -> ()
                          n248 = local write "Data"(w466) -> ()
                          n249 = local write "OK"(w468) -> ()
                          "DPT INICIALES I" <- "Potencia inicial lente izquierdo"
                        }
                      }
                      n250 = local read "Parar adquisicion"() -> (w447:bool)
                    }
                  }
                  frame Error {
                  }
                }
                n251 = VISA Close(VISA resource name=w342, error in (no error)=w343) -> (error out=w345:errorcluster)
                n252 = call <vilib>:"Simple Error Handler.vi"("error in (no error)"=w345) -> ("error out"=→"error out 4":errorcluster)  [unwired: 4 in, 4 out]
              }
              frame 1 {
                # "Mensaje que pregunta si desea realizar el experimento\ncon un nuevo usuario o con el actual"
                # "Se vuelven 0 los valores del WL y de la potencia óptica y distancia"
                # "En esta opcion se activa el modo experimento"
                n253 = property on="Waveform length" class="WFChart (strict)"("History Data"=dbl[][] [[0.0]]) -> ()  [unwired: 2 in, 2 out]
                n254 = property on="Potencia optica y distancia" class="WFChart (strict)"("History Data"=dbl[][] [[0.0]]) -> ()  [unwired: 2 in, 2 out]
                n255 = Two Button Dialog(message="Con quien desea realizar los experimentos?", 1:"Nuevo voluntario" ("F button name (\"Cancel\")"), 2:"Voluntario actual" ("T button name (\"OK\")")) -> (T button?=w506:bool)
                n256 = flat-sequence {
                  tunnel: w506 -> [w519]
                  tunnel: [w518] -> w504
                  tunnel: w503 -> [w518]
                  tunnel: [w511] -> w491
                  tunnel: w490 -> [w511]
                  tunnel: [w529] -> w507
                  tunnel: [w531] -> w505
                  tunnel: w504 -> [w531]
                  tunnel: [w530] -> w501
                  tunnel: w500 -> [w530]
                  tunnel: [w528] -> w492
                  tunnel: w491 -> [w528]
                  tunnel: w507 -> [w543]
                  tunnel: w505 -> [w542]
                  tunnel: [w541] -> w502
                  tunnel: w501 -> [w540]
                  tunnel: [w539] -> w498
                  tunnel: [w538] -> w497
                  tunnel: [w537] -> w495
                  tunnel: [w536] -> w493
                  tunnel: w492 -> [w536]
                  tunnel: w498 -> [w595]
                  tunnel: w497 -> [w578]
                  tunnel: [w595] -> w496
                  tunnel: w495 -> [w581]
                  tunnel: [w569] -> w494
                  tunnel: w493 -> [w569]
                  tunnel: [w598] -> w499
                  tunnel: w496 -> [w598]
                  tunnel: w494 -> [w596]
                  frame #0 {
                    # "Se guardan los datos de un nuevo voluntario"
                    n257 = Not(x=w519) -> (.not. x?=w513:bool)
                    n258 = case shown="True" w513 {
                      tunnel: [w522 w527] -> w517
                      tunnel: [w521 w526] -> w516
                      tunnel: [w523 w525] -> w515
                      tunnel: [w520 w524] -> w514
                      frame False {
                        n259 = local read "Enfermedad visual"() -> (w522:string)
                        n260 = local read "Nombre"() -> (w523:string)
                        n261 = local read "Cedula"() -> (w520:string)
                        n262 = local read "Edad"() -> (w521:string)
                      }
                      frame True {
                        n263 = call "Registro voluntario"() -> ("Enfermedad visual"=w527:string, "Edad"=w526:string, "Cedula"=w524:string, "Nombre"=w525:string)  [unwired: 14 in, 2 out]
                      }
                    }
                    "Cedula" <- w514
                    "Nombre" <- w515
                    "Edad" <- w516
                    "Enfermedad visual" <- w517
                    n264 = local write "T button?"(FALSE ("T button?")) -> ()
                  }
                  frame #1 {
                    n265 = Two Button Dialog(message="Qué tipo de experimento desea realizar?", 1:"Nuevo Experimento" ("F button name (\"Cancel\")"), 2:"Experimento existente" ("T button name (\"OK\")")) -> (T button?=w532:bool)
                    n266 = Not(x=w532) -> (.not. x?=w529:bool)
                  }
                  frame #2 {
                    # "A partir de la seleccion del experimento, se obtiene la descripcion correspondiente que será guardada en el archivo"
                    n267 = case shown="False" w543 {
                      tunnel: w542 -> [w545 w563]
                      tunnel: [w545 w562] -> w541
                      tunnel: w540 -> [w547 w561]
                      tunnel: [w547 w560] -> w539
                      tunnel: [w548 w559] -> w538
                      tunnel: [w544 w558] -> w537
                      frame False {
                        n268 = call "Display Message to User"() -> ()  [unwired: 10 in, 2 out]
                        n269 = flat-sequence {
                          tunnel: [w549] -> w546
                          tunnel: w545 -> [w549]
                          tunnel: [w557] -> w548
                          tunnel: w547 -> [w556]
                          tunnel: ["Menu experimentos"] -> _
                          tunnel: w546 -> [w554]
                          tunnel: [w553] -> w544
                          frame #0 {
                            n270 = while {
                              stop <- w550 stop-if-true
                              # "El sistema se queda en el loop hasta que el usuario elija el experimento que desea realizar"
                              n271 = event shown="[0] \"Elegir menu Exp\": Value Change" {
                                selector: _ -> [_ _]
                                dyn-events: _ -> [_ _]
                                timeout: _ -> [_ _]
                                tunnel: [TRUE FALSE] -> w550
                                event "Elegir menu Exp": Value Change {
                                n272 = event-data() -> ()  [unwired: 1 in, 4 out]
                                }
                                event Timeout {
                                n273 = event-data() -> ()  [unwired: 1 in, 3 out]
                                }
                              }
                            }
                          }
                          frame #1 {
                            n274 = Index Array(array=w556, index="Menu experimentos") -> (element=w557:string)
                            n275 = Index Array(array=w554, index="Menu experimentos") -> (element=w553:string)
                          }
                        }
                        "Array" <- w545
                      }
                      frame True {
                        # "Se añade el nuevo experimento al menu de seleccion de experimentos"
                        # "Se guarda el nuevo experimento en el archivo que los contiene"
                        n276 = call "Nuevo experimento"() -> ("Descripcion"=w559:string, "Nombre"=w558:string)  [unwired: 16 in, 2 out]
                        n277 = Insert Into Array(array=w561, new element=w559) -> (w560:string[])  [unwired: 1 in]
                        n278 = Insert Into Array(array=w563, new element=w558) -> (w562:string[])  [unwired: 1 in]
                        n279 = property on="Menu experimentos" class="Ring (strict)"("Strings []"=w562) -> ()  [unwired: 2 in, 2 out]
                        n280 = Insert Into Array(array=string[] [], new element #1=w558, new element #2=w559) -> (w565:string[])  [unwired: 1 in]
                        n281 = call-poly <vilib>:"Write Delimited Spreadsheet.vi"("file path (dialog if empty)"=path "C:/Users/TGM1603/Documents/LabVIEW Data/Experimentos_realizados", "1D data"=w565, "append to file? (new file:F)"=TRUE) -> ()  [unwired: 11 in, 2 out]
                      }
                    }
                  }
                  frame #3 {
                    # "Se guardan los datos generales del experimento en el archivo de excel"
                    n282 = local read "Frecuencia muestreo"() -> (w571:i32)
                    n283 = local read "factor decimacion"() -> (w577:i32)
                    n284 = local read "Enfermedad visual"() -> (w580:string)
                    n285 = local read "Cedula"() -> (w582:string)
                    n286 = local read "Edad"() -> (w579:string)
                    n287 = local read "Nombre"() -> (w583:string)
                    n288 = Get Date/Time In Seconds() -> (seconds since 1Jan1904=w594:timestamp)
                    n289 = Path To String(path="Carpeta") -> (string=w590:string)
                    n290 = Format Date/Time String(time format string (%c)="_%d-%m-%y_%H-%M", seconds (now)=w594) -> (date/time string=w592:string)  [unwired: 1 in]
                    n291 = Number To Fractional String(number=0.0, precision (6)=i16 0) -> (F-format string=w574:string)  [unwired: 2 in]
                    n292 = Number To Fractional String(number=w577, precision (6)=i16 0) -> (F-format string=w576:string)  [unwired: 2 in]
                    n293 = local read "Cedula"() -> (w586:string)
                    n294 = Number To Fractional String(number=w571, precision (6)=i16 0) -> (F-format string=w572:string)  [unwired: 2 in]
                    n295 = Concatenate Strings(w590, "\\" ("string"), w586, w592, "_" ("string"), w581, ".xlsx" ("string")) -> (w588:string)
                    n296 = String To Path(string=w588) -> (path=w587:path)
                    "path" <- w587
                    n297 = call "MS Office Report"("Path to Save Report"=w587, "Cedula"=w582, "decimacion"=w576, "Edad"=w579, "Enfermedad"=w580, "Exp_nombre"=w581, "Experimento"=w578, "freq"=w572, "Nombre"=w583, "rango"=w574) -> ()  [unwired: 16 in, 2 out]
                    "Nombre 2" <- w581
                  }
                  frame #4 {
                    n298 = while {
                      shift-right: [w600] -> _
                      shift-left: enum16{"Inicio", "Tomar datos", ""}."Inicio" -> [w602]
                      tunnel: w596 -> [w599]
                      stop <- w601 stop-if-true
                      n299 = case shown="\"Tomar datos\"" w602 {
                        tunnel: [w603 w614] -> w600
                        tunnel: w599 -> [_ w609]
                        frame "Inicio", Default {
                          # "Se chequea si el usuario ha presionado el boton de comenzar el experimento. Si no lo ha hecho, se queda en este estado (0).\n Cuando lo presiona, pasa al estado de adquirir datios (1) ."
                          n300 = Select(t=enum16{"Inicio", "Tomar datos", ""}."Tomar datos", s="Iniciar experimento", f=enum16{"Inicio", "Tomar datos", ""}."Inicio") -> (s? t:f=w603:enum16{"Inicio", "Tomar datos", ""})
                        }
                        frame "Tomar datos" {
                          n301 = flat-sequence {
                            tunnel: [w707] -> w613
                            tunnel: [w706] -> w612
                            tunnel: [w705] -> w611
                            tunnel: [w704] -> w610
                            tunnel: w609 -> [w698]
                            tunnel: [w681] -> w608
                            tunnel: [w661] -> w607
                            tunnel: w613 -> [w1014]
                            tunnel: w612 -> [w1013]
                            tunnel: w611 -> [w1012]
                            tunnel: w610 -> [w1011]
                            tunnel: w608 -> [w1008]
                            tunnel: w607 -> [w1009]
                            tunnel: [enum16{"Inicio", "Tomar datos", ""}."Inicio"] -> w614
                            frame #0 {
                              w618 = 10123 items=["Finite Samples"=10178, "Continuous Samples"=10123, "Hardware Timed Single Point"=12522] ("sample mode")
                              w622 = 10083 items=["Default"=-1, "RSE"=10083, "NRSE"=10078, "Differential"=10106, "Pseudodifferential"=12529] ("input terminal configuration")
                              w647 = u16 0 items=["None", "Last Bit", "TermChar", "Break"] ("Serial Settings:End Mode for Writes")
                              w648 = u16 2 items=["None", "Last Bit", "TermChar"] ("Serial Settings:End Mode for Reads")
                              w672 = u16 0 items=["None", "Last Bit", "TermChar", "Break"] ("Serial Settings:End Mode for Writes")
                              w673 = u16 2 items=["None", "Last Bit", "TermChar"] ("Serial Settings:End Mode for Reads")
                              w696 = 100  # max queue size
                              # "[9] Se unen en una sola matriz los vectores de tiempo, distancia, potencia derecha y potencia izquierda."
                              # "[9]"
                              # "[12] Se unen en una sola matriz, los vectores de  tiempo de la señal EMG, amplitud de la señal EMG, tiempo de potencia óptica, distancia, potencia óptica derecha y potencia óptica izquierda, en ese orden."
                              # "[8]"
                              # "[7]"
                              # "[6]"
                              # "[5]"
                              # "Se usan registros de desplazamiento para concatenar en un solo vector los datos que se obtienen en cada iteracion. Así en \n[1] Se guarda la potencia del lente derecho.\n[2] Por medio de variables locales, se guarda la distancia que se obtuvo en el bloque de distancia.\n[3]  Por medio de variables locales, se guarda la potencia del lente izquierdo que se obtuvo en el bloque de control de potencia del lente izquierdo.\n[4] Se guarda el tiempo actual.\n[5] Se pasa el vector de de potencia derecha a variable a string con 2 cifras significativas. \n[6] Se ajusta el vector del tiempo para que se muestre un tiempo relativo, es decir, en donde el primer dato sea 0 y en los demas se aumente un dt.  Además, se pasa el vector a variable a string con 5 cifras significativas.\n[7] Se pasa el vector de de distancia a variable a string con 0 cifras significativas. \n[8] Se pasa el vector de de potencia izquierda a variable a string con 2 cifras significativas."
                              # "En esta cola se guarda los datos de la señal EMG\nEn el bloque de adquisición los añade al adquirirlos y  en el de procesamiento los elimina al procesarlos ."
                              # "Initialize VISA port with correct parameters"
                              # "Initialize VISA port with correct parameters"
                              # "Close VISA port after program stop. Otherwise this port is blocked."
                              # "Se adquiere la señal del circuito de adquisicion, en donde se define la frecuencia de muestreo y el factor de decimacion.\n[1] Se inicializa el canal de adquisicion\n[2] Se ajusta el canal para que lea muestras continuas y apartir de estas prooduzca waveform data.\n[3]  Se obtiene los datos de la señal: la amplitud Y, el tiempo de inicio y el delta t.\n[4] Se decima el vector de amplitud. \n[5] Se usan registros de desplazamiento para concatenenar en un solo vector los datos de la amplitud que se obtienen en cada iteración. \n[6] Se obtiene el vector del tiempo."
                              # "[11] Los vectores de amplitud y tiempo se transforman a formato texto con 4 y 5 cifras significativas respectivamente y se unen para formar un vector de 2 columnas."
                              # "[9] Se ajusta el vector del tiempo para que se muestre un tiempo relativo, es decir, en donde el primer dato sea 0 y en los demas se aumente un dt. \n[10] Se extrae el primer elemento del vector ya que este siempre es 0 y no aporta información"
                              # "[12]"
                              # "[11]"
                              # "[10]"
                              # "[9]"
                              # "[8] Se guarda la fecha/hora en que se inicio el experimento"
                              # "[7] Se usan registros de desplazamiento para concatenar en un solo vector los datos del tiempo que se obtienen en cada iteracion."
                              # "[1]"
                              n302 = local read "error in (no error)"() -> (w668:errorcluster)
                              n303 = local read "VISA resource name"() -> (w667:string)
                              n304 = local read "VISA resource name 2"() -> (w643:string)
                              n305 = call-poly "VISA Configure Serial Port"("VISA resource name"=w667, "timeout (10sec)"=u32 2000, "Enable Termination\nChar (T)"=FALSE ("Enable Termination\nChar (T)"), "baud rate (9600)"=u32 115200, "error in (no error)"=w668) -> ("VISA resource name out"=w677:refnum<visa-resource-name>, "error out"=w675:errorcluster)  [unwired: 9 in]
                              n306 = call-poly "VISA Configure Serial Port"("VISA resource name"=w643, "timeout (10sec)"=u32 2000, "Enable Termination\nChar (T)"=FALSE ("Enable Termination\nChar (T)"), "baud rate (9600)"=u32 115200, "error in (no error)"="error in (no error) 5") -> ("VISA resource name out"=w652:refnum<visa-resource-name>, "error out"=w650:errorcluster)  [unwired: 9 in]
                              n307 = property class="Instr"(reference=w677, error in=w675, "TermChar"=u8 10 ("Message Based Settings:Termination Character"), "ASRL End In"=w673, "ASRL End Out"=w672) -> (reference out=w676:refnum<visa-resource-name>, error out=w674:errorcluster)
                              n308 = property class="Instr"(reference=w652, error in=w650, "TermChar"=u8 10 ("Message Based Settings:Termination Character"), "ASRL End In"=w648, "ASRL End Out"=w647) -> (reference out=w651:refnum<visa-resource-name>, error out=w649:errorcluster)
                              n309 = VISA Set I/O Buffer Size(VISA resource name=w676, error in (no error)=w674) -> (VISA resource name out=w670:refnum<visa-resource-name>, error out=w669:errorcluster)  [unwired: 2 in]
                              n310 = VISA Set I/O Buffer Size(VISA resource name=w651, error in (no error)=w649) -> (VISA resource name out=w645:refnum<visa-resource-name>, error out=w644:errorcluster)  [unwired: 2 in]
                              n311 = VISA Flush I/O Buffer(VISA resource name=w670, error in (no error)=w669) -> (VISA resource name out=w666:refnum<visa-resource-name>, error out=w665:errorcluster)  [unwired: 1 in]
                              n312 = call-poly <vilib>:"DAQmx Create Virtual Channel.vi"("input terminal configuration"=w622, "physical channels"=tag "Dev1/ai0") -> ("task out"=w621:refnum<k21>, "error out"=w620:errorcluster)  [unwired: 12 in]
                              n313 = VISA Flush I/O Buffer(VISA resource name=w645, error in (no error)=w644) -> (VISA resource name out=w641:refnum<visa-resource-name>, error out=w640:errorcluster)  [unwired: 1 in]
                              n314 = invoke on="Parar adquisicion" class="Bool (strict)" method="Reinit To Default"() -> ()  [unwired: 3 in, 3 out]
                              n315 = Obtain Queue(max queue size (-1, unlimited)=w696, element data type="Cola tipo 2") -> (queue out=w695:refnum<queue>)  [unwired: 3 in, 2 out]
                              n316 = Enqueue Element(queue=w698, element=0.0) -> (queue out=w701:refnum<queue>)  [unwired: 2 in, 2 out]
                              n317 = call-poly <vilib>:"DAQmx Timing.vi"("task/channels in"=w621, "sample mode"=w618, "samples per channel"=1000, "rate"=1000.0, "error in"=w620) -> ("task out"=w616:refnum<k21>, "error out"=w615:errorcluster)  [unwired: 9 in]
                              n318 = call <vilib>:"DAQmx Start Task.vi"("task/channels in"=w616, "error in"=w615) -> ("task out"=w720:refnum<k21>, "error out"=w721:errorcluster)  [unwired: 12 in]
                              n319 = local read "tamaño buffer"() -> (w719:i32)
                              n320 = case shown="No Error" w640 {
                                tunnel: w640 -> [w744 w801]
                                tunnel: w641 -> [w743 w802]
                                tunnel: [w742 w801] -> w627
                                tunnel: [w741 w802] -> w626
                                tunnel: [w731 dbl[] [-30.0]] -> _
                                frame No Error {
                                w740 = 2 ("length (rest)")
                                # "Bloque de control del izquierdo. Se explica en el caso 0 de visualziación general"
                                # "Initialize Lens Driver"
                                n321 = local read "Calibration"() -> (w732:T2)
                                n322 = for {
                                tunnel: w743 -> [w798]
                                tunnel: [w795] -> w735
                                tunnel: string[] ["Start", "MwDA", "CrMA00", "CrMB00", "CrUA00", "CrUB00", "CrLA00", "CrLB00", "PwTA\u0002Ð\u0001@"] -> [w793] mode=indexing
                                tunnel: [w792] -> w734
                                shift-right: [w796] -> w736
                                shift-left: w732 -> [w797]
                                shift-right: [w794] -> w737
                                shift-left: w744 -> [w799]
                                n323 = call "write read Lens Driver.vi"("VISA resource name"=w798, "command"=w793, "Calibration"=w797, "error in (no error)"=w799) -> ("VISA resource name out"=w795:refnum<visa-resource-name>, "Calibration 2"=w796:T2, "Data"=w792:string, "error out"=w794:errorcluster)  [unwired: 4 in, 4 out]
                                }
                                n324 = String Subset(string=w734, offset (0)=w740, length (rest)=w740) -> (substring=w738:string)
                                n325 = Type Cast(type=u16 0 ("length (rest)"), x=w738) -> (*(type *) &x=w733:u16)
                                n326 = local write "ID"(w733) -> ()
                                n327 = while {
                                tunnel: [w749] -> w742
                                tunnel: [w750] -> w741
                                tunnel: w737 -> [w755]
                                tunnel: w736 -> [w754]
                                tunnel: w735 -> [w753]
                                shift-right: [w746] -> w731
                                shift-left: _ -> [w747]
                                stop <- w748 stop-if-true
                                # "When Send command is true, Current Ch A is sent to the Lens Driver, in the correct format. If answer exists it is displayed in Data. The update rate of the while loop is 2ms."
                                n328 = case shown="True" TRUE ("Send command") {
                                tunnel: [w761 w784] -> w749
                                tunnel: w755 -> [w761 w783]
                                tunnel: w754 -> [_ w764]
                                tunnel: w753 -> [w760 w782]
                                tunnel: [w760 w775] -> w750
                                tunnel: [dbl[] [-20.0] w774] -> w746
                                tunnel: w747 -> [_ w773]
                                frame False {
                                }
                                frame True {
                                n329 = local read "Potencia inicial lente izquierdo"() -> (w772:dbl)
                                n330 = local read "DPT dif."() -> (w771:dbl)
                                n331 = Add(x=w771, y=w772) -> (x+y=w767:dbl)
                                n332 = Absolute Value(x=w767) -> (abs(x)=w769:dbl)
                                n333 = Greater Or Equal?(x=6.0, y=w769) -> (x >= y?=w768:bool)
                                n334 = case shown="False" w768 {
                                tunnel: w767 -> [w787 w791]
                                tunnel: [w785 w791] -> w765
                                frame False {
                                n335 = Greater Or Equal?(x=u16 0, y=w787) -> (x >= y?=w788:bool)
                                n336 = case shown="False" w788 {
                                tunnel: [i16 6 ("x") i16 -6 ("x")] -> w785
                                frame False {
                                }
                                frame True {
                                }
                                }
                                }
                                frame True {
                                }
                                }
                                "Potencia izquierdo" <- w765
                                n337 = Unbundle By Name(w764) -> ("Max Current A"=w763:dbl)
                                n338 = call "potencia a corriente.vi"("Max current A"=w763, "Potencia"=w765) -> ("Corriente"=w766:dbl)
                                n339 = To Word Integer(number=w766) -> (16bit integer=w781:i16)
                                n340 = Type Cast(x=w781) -> (*(type *) &x=w780:string)  [unwired: 1 in]
                                n341 = Concatenate Strings("Aw", w780) -> (w777:string)
                                n342 = local write "Command to Port"(w777) -> ()
                                n343 = call "write read Lens Driver.vi"("VISA resource name"=w782, "command"=w777, "Calibration"=w764, "error in (no error)"=w783) -> ("VISA resource name out"=w775:refnum<visa-resource-name>, "Calibration 2"=w779:T2, "OK"=w778:bool, "Data"=w776:string, "error out"=w784:errorcluster)  [unwired: 4 in, 3 out]
                                n344 = local write "VISA resource name 2"(w775) -> ()
                                n345 = local write "Calibration 2"(w779) -> ()
                                n346 = local write "Data"(w776) -> ()
                                n347 = local write "OK"(w778) -> ()
                                n348 = Build Array (concatenate)(w773, w765) -> (w774:dbl[])
                                }
                                }
                                n349 = Wait Until Next ms Multiple(millisecond multiple=u32 10) -> ()  [unwired: 1 out]
                                n350 = local read "Parar adquisicion"() -> (w748:bool)
                                n351 = event shown="[0] \"Restablecer Iniciales\": Value Change" {
                                selector: _ -> [_ _]
                                dyn-events: _ -> [_ _]
                                timeout: 100 -> [_ _]
                                event "Restablecer Iniciales": Value Change {
                                n352 = event-data() -> ()  [unwired: 1 in, 3 out]
                                n353 = local read "Potencia inicial lente izquierdo"() -> (w756:dbl)
                                n354 = local read "Potencia inicial lente derecho"() -> (w757:dbl)
                                n355 = local write "Potencia izquierdo"(w756) -> ()
                                n356 = local write "Potencia derecho"(w757) -> ()
                                n357 = local write "DPT dif."(0.0 ("DPT dif.")) -> ()
                                }
                                event Timeout {
                                n358 = event-data() -> ()  [unwired: 1 in, 3 out]
                                }
                                }
                                }
                                }
                                frame Error {
                                }
                              }
                              n359 = case shown="No Error" w665 {
                                tunnel: w665 -> [w824 w920]
                                tunnel: w666 -> [w823 w921]
                                tunnel: [w822 w920] -> w693
                                tunnel: [w821 w921] -> w692
                                tunnel: [w810 dbl[] [-1.0]] -> w685
                                tunnel: [w809 dbl[] [-30.0]] -> w633
                                tunnel: [w808 u32[] [0]] -> w663
                                tunnel: [w806 dbl[] [-30.0]] -> w636
                                frame No Error {
                                w820 = 2 ("length (rest)")
                                # "Bloque de control del lente derecho. Se explica en el caso 0 de visualziación general"
                                # "Initialize Lens Driver"
                                n360 = local read "Calibration"() -> (w812:T2)
                                n361 = for {
                                tunnel: w823 -> [w914]
                                tunnel: [w911] -> w815
                                tunnel: string[] ["Start", "MwDA", "CrMA00", "CrMB00", "CrUA00", "CrUB00", "CrLA00", "CrLB00", "PwTA\u0002Ð\u0001@"] -> [w909] mode=indexing
                                tunnel: [w908] -> w814
                                shift-right: [w912] -> w816
                                shift-left: w812 -> [w913]
                                shift-right: [w910] -> w817
                                shift-left: w824 -> [w915]
                                n362 = call "write read Lens Driver.vi"("VISA resource name"=w914, "command"=w909, "Calibration"=w913, "error in (no error)"=w915) -> ("VISA resource name out"=w911:refnum<visa-resource-name>, "Calibration 2"=w912:T2, "Data"=w908:string, "error out"=w910:errorcluster)  [unwired: 4 in, 4 out]
                                }
                                n363 = String Subset(string=w814, offset (0)=w820, length (rest)=w820) -> (substring=w818:string)
                                n364 = Type Cast(type=u16 0 ("length (rest)"), x=w818) -> (*(type *) &x=w813:u16)
                                n365 = local write "ID"(w813) -> ()
                                n366 = while {
                                tunnel: [w842] -> w822
                                tunnel: [w843] -> w821
                                tunnel: w817 -> [w848]
                                tunnel: w816 -> [w847]
                                tunnel: w815 -> [w846]
                                shift-right: [w829] -> w810
                                shift-left: dbl[] [0.0] -> [w830]
                                shift-right: [w837] -> w809
                                shift-left: dbl[] [0.0] -> [w840]
                                shift-right: [w836] -> w808
                                shift-left: u32[] [0] -> [w839]
                                shift-right: [w827] -> w806
                                shift-left: dbl[] [0.0] -> [w826]
                                stop <- w841 stop-if-true
                                # "[4]"
                                # "[3]"
                                # "[2]"
                                # "When Send command is true, Current Ch A is sent to the Lens Driver, in the correct format. If answer exists it is displayed in Data. The update rate of the while loop is 2ms."
                                n367 = Wait Until Next ms Multiple(millisecond multiple=u32 10) -> ()  [unwired: 1 out]
                                n368 = case shown="True" TRUE ("Send command") {
                                tunnel: [w855 w874] -> w842
                                tunnel: w848 -> [w855 w873]
                                tunnel: w847 -> [_ w858]
                                tunnel: w846 -> [w854 w872]
                                tunnel: [w854 w864] -> w843
                                tunnel: [dbl[] [-20.0] w863] -> w837
                                tunnel: w840 -> [_ w862]
                                frame False {
                                }
                                frame True {
                                # "[1]"
                                n369 = local read "number"() -> (w869:u32)
                                n370 = local read "Potencia inicial lente derecho"() -> (w861:dbl)
                                n371 = case shown="2" w869 {
                                tunnel: [w875 w884 w899] -> w860
                                tunnel: w861 -> [w877 w879 w894]
                                tunnel: w861 -> [_ w878 w893]
                                frame 0, Default {
                                n372 = local read "DPT dif."() -> (w876:dbl)
                                n373 = Add(x=w877, y=w876) -> (x+y=w875:dbl)
                                }
                                frame 1 {
                                n374 = local read "DPT dif."() -> (w880:dbl)
                                n375 = Add(x=w879, y=w880) -> (x+y=w881:dbl)
                                n376 = Less Or Equal?(x=w881, y=6.0) -> (x <= y?=w883:bool)
                                n377 = case shown="True" w883 {
                                tunnel: [w886 w890] -> w884
                                tunnel: w878 -> [w885 w889]
                                frame False {
                                n378 = local read "DPT dif."() -> (w887:dbl)
                                n379 = Add(x=w885, y=w887) -> (x+y=w886:dbl)
                                }
                                frame True {
                                n380 = local read "DPT dif."() -> (w891:dbl)
                                n381 = local read "Incremento"() -> (w888:dbl)
                                n382 = Add(x=w891, y=w888) -> (x+y=w892:dbl)
                                n383 = local write "DPT dif."(w892) -> ()
                                n384 = Add(x=w889, y=w892) -> (x+y=w890:dbl)
                                }
                                }
                                }
                                frame 2 {
                                n385 = local read "DPT dif."() -> (w898:dbl)
                                n386 = Add(x=w898, y=w894) -> (x+y=w895:dbl)
                                n387 = Greater Or Equal?(x=w895, y=-6.0) -> (x >= y?=w896:bool)
                                n388 = case shown="True" w896 {
                                tunnel: [w901 w905] -> w899
                                tunnel: w893 -> [w900 w904]
                                frame False {
                                n389 = local read "DPT dif."() -> (w902:dbl)
                                n390 = Add(x=w900, y=w902) -> (x+y=w901:dbl)
                                }
                                frame True {
                                n391 = local read "DPT dif."() -> (w907:dbl)
                                n392 = local read "Incremento"() -> (w903:dbl)
                                n393 = Subtract(x=w907, y=w903) -> (x-y=w906:dbl)
                                n394 = local write "DPT dif."(w906) -> ()
                                n395 = Add(x=w904, y=w906) -> (x+y=w905:dbl)
                                }
                                }
                                }
                                }
                                "Potencia derecho" <- w860
                                n396 = Unbundle By Name(w858) -> ("Max Current A"=w857:dbl)
                                n397 = call "potencia a corriente.vi"("Max current A"=w857, "Potencia"=w860) -> ("Corriente"=w859:dbl)
                                n398 = To Word Integer(number=w859) -> (16bit integer=w871:i16)
                                n399 = Type Cast(x=w871) -> (*(type *) &x=w870:string)  [unwired: 1 in]
                                n400 = Concatenate Strings("Aw", w870) -> (w866:string)
                                n401 = local write "Command to Port"(w866) -> ()
                                n402 = call "write read Lens Driver.vi"("VISA resource name"=w872, "command"=w866, "Calibration"=w858, "error in (no error)"=w873) -> ("VISA resource name out"=w864:refnum<visa-resource-name>, "Calibration 2"=w868:T2, "OK"=w867:bool, "Data"=w865:string, "error out"=w874:errorcluster)  [unwired: 4 in, 3 out]
                                n403 = local write "VISA resource name out"(w864) -> ()
                                n404 = local write "Calibration 2"(w868) -> ()
                                n405 = local write "Data"(w865) -> ()
                                n406 = local write "OK"(w867) -> ()
                                n407 = Build Array (concatenate)(w862, w860) -> (w863:dbl[])
                                }
                                }
                                n408 = local read "Parar adquisicion"() -> (w841:bool)
                                n409 = local read "Potencia izquierdo"() -> (w825:dbl)
                                n410 = local read "Distancia"() -> (w838:u32)
                                n411 = property on="Potencia optica y distancia" class="WFChart (strict)"("YScale.ScaleFit"="Auto scale Y") -> ()  [unwired: 2 in, 2 out]
                                n412 = Get Date/Time In Seconds() -> (seconds since 1Jan1904=w831:timestamp)
                                n413 = To Double Precision Float(number=w831) -> (double precision float=w828:dbl)
                                n414 = property on="Potencia optica y distancia" class="WFChart (strict)"("XScale.ScaleFit"="Auto scale X") -> ()  [unwired: 2 in, 2 out]
                                n415 = Build Array (concatenate)(w830, w828) -> (w829:dbl[])
                                n416 = case shown="0, Default" "Auto scale Y" {
                                frame 0, Default {
                                n417 = property on="Potencia optica y distancia" class="WFChart (strict)"("YScale.Maximum"="Escala Y max") -> ()  [unwired: 2 in, 2 out]
                                n418 = property on="Potencia optica y distancia" class="WFChart (strict)"("YScale.Minimum"="Escala Y min") -> ()  [unwired: 2 in, 2 out]
                                }
                                frame 1 {
                                }
                                }
                                n419 = Build Array (concatenate)(w826, w825) -> (w827:dbl[])
                                n420 = Build Array (concatenate)(w839, w838) -> (w836:u32[])
                                n421 = case shown="0, Default" "Auto scale X" {
                                frame 0, Default {
                                n422 = property on="Potencia optica y distancia" class="WFChart (strict)"("XScale.Maximum"="Escala X max") -> ()  [unwired: 2 in, 2 out]
                                n423 = property on="Potencia optica y distancia" class="WFChart (strict)"("XScale.Minimum"="Escala X min") -> ()  [unwired: 2 in, 2 out]
                                }
                                frame 1 {
                                }
                                }
                                n424 = Build Array(w837, w836) -> (w835:dbl[][])
                                n425 = Transpose 2D Array(2D array=w835) -> (transposed array=→"Potencia optica y distancia":dbl[][])
                                }
                                }
                                frame Error {
                                }
                              }
                              n426 = while {
                                tunnel: w701 -> [w953]
                                shift-right: [w955] -> _
                                shift-left: dbl[] [0.0] -> [w961]
                                shift-right: [w954] -> _
                                shift-left: u32[] [0] -> [w956]
                                tunnel: [w953] -> w699
                                tunnel: w695 -> [w945]
                                stop <- w944 stop-if-true
                                # "Bloque de procesamiento.  Se explica en el caso 0 de visualización general"
                                n427 = local read "WL"() -> (w952:dbl)
                                n428 = local read "Parar adquisicion"() -> (w944:bool)
                                n429 = local read "Limite superior WL"() -> (w949:dbl)
                                n430 = call "waveform_length.vi"("WL"=w952, "Cola WL"=w953, "Datos entrada"=w945) -> ("WL 2"=w960:dbl)
                                n431 = local read "Limite inferior WL"() -> (w951:dbl)
                                n432 = local write "WL"(w960) -> ()
                                n433 = Build Array (concatenate)(w961, w960) -> (w955:dbl[])
                                n434 = In Range and Coerce(upper limit=w949, x=w960, lower limit=w951) -> (In Range?=w958:bool)  [unwired: 1 out]
                                n435 = Greater?(x=w960, y=w949) -> (0:w959:bool)
                                n436 = local read "Escala autom. X"() -> (w946:u8)
                                n437 = local read "Escala autom. Y"() -> (w947:u8)
                                n438 = Build Array(w959, w958) -> (w957:bool[])
                                n439 = Boolean Array To Number(Boolean array=w957) -> (number=w950:u32)
                                n440 = local write "number"(w950) -> ()
                                n441 = Build Array (concatenate)(w956, w950) -> (w954:u32[])
                                n442 = Build Array(w955, w954) -> (w948:dbl[][])
                                n443 = Transpose 2D Array(2D array=w948) -> (transposed array=w943:dbl[][])
                                n444 = local write "Waveform length"(w943) -> ()
                                n445 = property on="Waveform length" class="WFChart (strict)"("XScale.ScaleFit"=w946) -> ()  [unwired: 2 in, 2 out]
                                n446 = property on="Waveform length" class="WFChart (strict)"("YScale.ScaleFit"=w947) -> ()  [unwired: 2 in, 2 out]
                                n447 = case shown="0, Default" w947 {
                                frame 0, Default {
                                n448 = local read "Maximo escala Y"() -> (w965:dbl)
                                n449 = local read "Minimo escala Y"() -> (w964:dbl)
                                n450 = property on="Waveform length" class="WFChart (strict)"("YScale.Maximum"=w965) -> ()  [unwired: 2 in, 2 out]
                                n451 = property on="Waveform length" class="WFChart (strict)"("YScale.Minimum"=w964) -> ()  [unwired: 2 in, 2 out]
                                }
                                frame 1 {
                                }
                                }
                                n452 = case shown="0, Default" w946 {
                                frame 0, Default {
                                n453 = local read "Minimo escala X"() -> (w963:dbl)
                                n454 = local read "Maximo escala X"() -> (w962:dbl)
                                n455 = property on="Waveform length" class="WFChart (strict)"("XScale.Minimum"=w963) -> ()  [unwired: 2 in, 2 out]
                                n456 = property on="Waveform length" class="WFChart (strict)"("XScale.Maximum"=w962) -> ()  [unwired: 2 in, 2 out]
                                }
                                frame 1 {
                                }
                                }
                              }
                              n457 = while {
                                tunnel: w720 -> [w998]
                                tunnel: w719 -> [w995]
                                tunnel: [w996] -> w709
                                shift-right: [w993] -> w708
                                shift-left: w721 -> [w997]
                                tunnel: [w988] -> w729
                                shift-right: [w987] -> w706
                                shift-left: _ -> [w986]
                                shift-right: [w977] -> w711
                                shift-left: dbl[] [0.0] -> [w982]
                                shift-right: [w978] -> w716
                                shift-left: dbl[] [0.0] -> [w979]
                                tunnel: w695 -> [w970]
                                i -> [w989]
                                stop <- w992 stop-if-true
                                w991 = 10.0  # timeout (s)
                                # "[7]"
                                # "[6]"
                                # "[5]"
                                # "[4]"
                                # "[3]"
                                # "[2]"
                                n458 = local read "Escala automatica X"() -> (w968:u8)
                                n459 = local read "Escala automatica Y"() -> (w967:u8)
                                n460 = property on="Senal EMG" class="WFGraph (strict)"("XScale.ScaleFit"=w968) -> ()  [unwired: 2 in, 2 out]
                                n461 = case shown="0, Default" w968 {
                                frame 0, Default {
                                n462 = local read "X Scale.Range:Increment"() -> (w1001:dbl)
                                n463 = local read "X Scale.Range:Minimum"() -> (w1002:dbl)
                                n464 = local read "X Scale.Range:Maximum"() -> (w1003:dbl)
                                n465 = property on="Senal EMG" class="WFGraph (strict)"("XScale.Increment"=w1001) -> ()  [unwired: 2 in, 2 out]
                                n466 = property on="Senal EMG" class="WFGraph (strict)"("XScale.Minimum"=w1002) -> ()  [unwired: 2 in, 2 out]
                                n467 = property on="Senal EMG" class="WFGraph (strict)"("XScale.Maximum"=w1003) -> ()  [unwired: 2 in, 2 out]
                                }
                                frame 1 {
                                }
                                }
                                n468 = local read "Parar adquisicion"() -> (w973:bool)
                                n469 = call-poly <vilib>:"DAQmx Read.vi"("task/channels in"=w998, "number of samples per channel"=w995, "timeout"=w991, "error in"=w997) -> ("task out"=w996:refnum<k21>, "data"=w983:waveform(dbl)[], "error out"=w993:errorcluster)  [unwired: 9 in]
                                n470 = Unbundle By Name(w993) -> ("status"=w994:bool)
                                n471 = Or(x=w994, y=w973) -> (x .or. y?=w992:bool)
                                n472 = property on="Senal EMG" class="WFGraph (strict)"("YScale.ScaleFit"=w967) -> ()  [unwired: 2 in, 2 out]
                                n473 = local write "Senal EMG"(w983) -> ()
                                n474 = case shown="0, Default" w967 {
                                frame 0, Default {
                                n475 = local read "Y Scale.Range:Maximum"() -> (w1000:dbl)
                                n476 = local read "Y Scale.Range:Minimum"() -> (w999:dbl)
                                n477 = property on="Senal EMG" class="WFGraph (strict)"("YScale.Minimum"=w999) -> ()  [unwired: 2 in, 2 out]
                                n478 = property on="Senal EMG" class="WFGraph (strict)"("YScale.Maximum"=w1000) -> ()  [unwired: 2 in, 2 out]
                                }
                                frame 1 {
                                }
                                }
                                n479 = call-poly <vilib>:"Index Waveform Array.vi"("index"=0, "waveform array"=w983) -> ("waveform"=w981:waveform(dbl))  [unwired: 8 in, 1 out]
                                n480 = Unbundle By Name(w981) -> ("Y"=w971:dbl[], "t0"=w988:timestamp)  [unwired: 1 out]
                                n481 = call-poly <vilib>:"Decimate (continuous).vi"("averaging"=TRUE, "decimating factor"="factor decimacion", "X"=w971) -> ("Decimated Array"=w966:dbl[])  [unwired: 7 in, 1 out]
                                n482 = Lossy Enqueue Element(queue=w970, element=w966) -> ()  [unwired: 1 in, 4 out]
                                n483 = Build Array (concatenate)(w982, w966) -> (w977:dbl[])
                                n484 = case shown="1" w989 {
                                tunnel: w988 -> [_ w1007]
                                tunnel: [w1005 w1006] -> w987
                                tunnel: w986 -> [w1005 _]
                                frame 0, Default {
                                }
                                frame 1 {
                                # "[8]"
                                n485 = Format Date/Time String(seconds (now)=w1007) -> (date/time string=w1006:string)  [unwired: 2 in]
                                }
                                }
                                n486 = local read "factor decimacion"() -> (w974:i32)
                                n487 = call-poly <vilib>:"Get Waveform Time Array.vi"("waveform in"=w981) -> ("X array"=w980:timestamp[])  [unwired: 9 in, 1 out]
                                n488 = event shown="[0] \"Ganancia\": Value Change" {
                                selector: _ -> [_ _]
                                dyn-events: _ -> [_ _]
                                timeout: 1 -> [_ _]
                                tunnel: "Ganancia" -> [w1004 _]
                                event "Ganancia": Value Change {
                                n489 = event-data() -> ()  [unwired: 1 in, 4 out]
                                n490 = call "Ganancia programable.vi"("MOSI data"=w1004) -> ()
                                }
                                event Timeout {
                                n491 = event-data() -> ()  [unwired: 1 in, 3 out]
                                }
                                }
                                n492 = To Double Precision Float(number=w980) -> (double precision float=w976:dbl[])
                                n493 = call-poly <vilib>:"Decimate (single shot).vi"("decimating factor"=w974, "X"=w976) -> ("Decimated Array"=w975:dbl[])  [unwired: 8 in, 1 out]
                                n494 = Build Array (concatenate)(w979, w975) -> (w978:dbl[])
                              }
                              n495 = call <vilib>:"DAQmx Clear Task.vi"("task in"=w709, "error in"=w708) -> ()  [unwired: 13 in, 1 out]
                              n496 = Index Array(array=w716, index=1) -> (element=w715:dbl)
                              n497 = Flush Queue(queue=w699) -> ()  [unwired: 1 in, 3 out]
                              n498 = Subtract(x=w716, y=w715) -> (x-y=w713:dbl[])
                              n499 = Delete From Array(array=w711, index=0) -> (array with subset deleted=w724:dbl[])  [unwired: 1 in, 1 out]
                              n500 = while {
                                shift-right: [w922] -> _
                                shift-left: _ -> [w923]
                                stop <- w927 stop-if-true
                                # "Este bloque adquiere la distancia (se explica en el caso 0 (visualizacion general)"
                                n501 = call "meididor de distancia archivo adicional.vi"() -> ("error out"=w930:errorcluster, "task out"=w931:refnum<k21>)  [unwired: 10 in]
                                n502 = call "DAQ Assistant2"("timeout (s)"=0.05) -> ("data"=w940:dynamicdata, "error out"=w928:errorcluster)  [unwired: 16 in, 1 out]
                                n503 = call <vilib>:"DAQmx Start Task.vi"("task/channels in"=w931, "error in"=w930) -> ("task out"=w934:refnum<k21>, "error out"=w935:errorcluster)  [unwired: 12 in]
                                n504 = call <vilib>:"DAQmx Is Task Done.vi"("task/channels in"=w934, "error in"=w935) -> ("task out"=w932:refnum<k21>, "error out"=w933:errorcluster)  [unwired: 11 in, 1 out]
                                n505 = Wait (ms)(milliseconds to wait=u32 200) -> ()  [unwired: 1 out]
                                n506 = call <vilib>:"Clear Errors.vi"("error in (no error)"=w928) -> ()  [unwired: 5 in, 2 out]
                                n507 = local read "Parar adquisicion"() -> (w927:bool)
                                n508 = call <vilib>:"DAQmx Clear Task.vi"("task in"=w932, "error in"=w933) -> ()  [unwired: 13 in, 1 out]
                                n509 = Multiply(x=1000000.0, y=w940) -> (x*y=w938:dynamicdata)
                                n510 = Divide(x=w938, y=58.0) -> (x/y=w924:dynamicdata)
                                n511 = Equal?(x=w924, y=0.0) -> (x = y?=w926:dynamicdata)
                                n512 = case shown="True" w926 {
                                tunnel: [w941 w942] -> w922
                                tunnel: w924 -> [w941 _]
                                tunnel: w923 -> [_ w942]
                                frame False {
                                }
                                frame True {
                                }
                                }
                                n513 = local write "Distancia"(w922) -> ()
                              }
                              n514 = Delete From Array(array=w713, index=0) -> (array with subset deleted=w723:dbl[])  [unwired: 1 in, 1 out]
                              n515 = local read "path"() -> (w707:path)
                              n516 = Format Date/Time String(seconds (now)=w729) -> (date/time string=w705:string)  [unwired: 2 in]
                              n517 = Number To Fractional String(use system decimal point (T)=FALSE, number=w724, precision (6)=i16 4) -> (F-format string=w659:string[])  [unwired: 1 in]
                              n518 = Number To Fractional String(use system decimal point (T)=FALSE, number=w723, precision (6)=i16 5) -> (F-format string=w660:string[])  [unwired: 1 in]
                              n519 = Build Array(w660, w659) -> (w722:string[][])
                              n520 = Transpose 2D Array(2D array=w722) -> (transposed array=w704:string[][])
                              n521 = Delete From Array(array=w633, index=0) -> (array with subset deleted=w632:dbl[])  [unwired: 1 in, 1 out]
                              n522 = Delete From Array(array=w663, index=0) -> (array with subset deleted=w629:u32[])  [unwired: 1 in, 1 out]
                              n523 = Index Array(array=w685, index=1) -> (element=w690:dbl)
                              n524 = Delete From Array(array=w636, index=0) -> (array with subset deleted=w635:dbl[])  [unwired: 1 in, 1 out]
                              n525 = VISA Close(VISA resource name=w626, error in (no error)=w627) -> (error out=w625:errorcluster)
                              n526 = Subtract(x=w685, y=w690) -> (x-y=w684:dbl[])
                              n527 = Number To Fractional String(use system decimal point (T)=FALSE, number=w632, precision (6)=i16 2) -> (F-format string=w656:string[])  [unwired: 1 in]
                              n528 = VISA Close(VISA resource name=w692, error in (no error)=w693) -> (error out=w694:errorcluster)
                              n529 = call <vilib>:"Simple Error Handler.vi"("error in (no error)"=w625) -> ("error out"=w624:errorcluster)  [unwired: 4 in, 4 out]
                              n530 = Number To Fractional String(number=w629, precision (6)=i16 0) -> (F-format string=w657:string[])  [unwired: 2 in]
                              n531 = Delete From Array(array=w684, index=0) -> (array with subset deleted=w689:dbl[])  [unwired: 1 in, 1 out]
                              n532 = call <vilib>:"Simple Error Handler.vi"("error in (no error)"=w694) -> ("error out"=w691:errorcluster)  [unwired: 4 in, 4 out]
                              n533 = Number To Fractional String(use system decimal point (T)=FALSE, number=w635, precision (6)=i16 2) -> (F-format string=w637:string[])  [unwired: 1 in]
                              n534 = local write "error out"(w691) -> ()
                              n535 = local write "error out"(w624) -> ()
                              n536 = Number To Fractional String(use system decimal point (T)=FALSE, number=w689, precision (6)=i16 5) -> (F-format string=w658:string[])  [unwired: 1 in]
                              n537 = Build Array(w660, w659, w658, w657, w656, w637) -> (w630:string[][])
                              n538 = Transpose 2D Array(2D array=w630) -> (transposed array=w661:string[][])
                              n539 = Build Array(w658, w657, w656, w637) -> (w681:string[][])
                            }
                            frame #1 {
                              # "[13]"
                              # "[13] En esta case structure, se decide que datos se van a guardar. Esto lo hace el SUBVI llamado guardar datos de amplitud y tiempo."
                              n540 = Transpose 2D Array(2D array=w1008) -> (transposed array=w1010:string[][])
                              n541 = call <vilib>:"Three Button Dialog.vi"("Right Button Text (\"Cancel\")"="Señal EMG, potencia optica y distancia" ("Right Button Text (\"Cancel\")"), "Center Button Text (\"No\")"="Potencia optica y distancia" ("Center Button Text (\"No\")"), "Left Button Text (\"Yes\")"="Señal EMG" ("Left Button Text (\"Yes\")"), "message"="Elija que datos desea guardar") -> ("Which Button?"=w1015:T3)  [unwired: 7 in]
                              n542 = case shown="\"Center Button\"" w1015 {
                                tunnel: w1014 -> [w1024 w1029 w1032]
                                tunnel: w1013 -> [w1023 w1028 w1033]
                                tunnel: w1012 -> [w1022 w1027 w1034]
                                tunnel: w1011 -> [w1021 _ _]
                                tunnel: w1010 -> [_ w1026 _]
                                tunnel: w1009 -> [_ _ w1030]
                                frame "Left Button", Default {
                                # "Se guarda solo la señal EMG y su tiempo de adquisición."
                                n543 = call "Guardar datos de Amplitud y Tiempo.vi"("path"=w1024, "Hora inicio"=w1023, "Hora fin"=w1022, "Datos experimento"=w1021, "column headers"=string[] ["Tiempo(s)", "Amplitud(V)"]) -> ()  [unwired: 1 in]
                                }
                                frame "Center Button" {
                                # "Se guarda la potenica del lente derecho, del lente izquierdo, la distancia y el tiempo de estas variables."
                                n544 = call "Guardar datos de Amplitud y Tiempo.vi"("path"=w1029, "Hora inicio"=w1028, "Hora fin"=w1027, "Datos experimento"=w1026, "column headers"=string[] ["Tiempo(s)", "Distancia (cm)", "Potencia Optica derecho", "Potencia optica izquierdo"]) -> ()  [unwired: 1 in]
                                }
                                frame "Right Button" {
                                # "Se guarda el tiempo de adquisición así como la amplitud de la señal EMG,  la potenica del lente derecho, del lente izquierdo, la distancia y el tiempo de estas variables."
                                n545 = call "Guardar datos de Amplitud y Tiempo.vi"("path"=w1032, "Hora inicio"=w1033, "Hora fin"=w1034, "Datos experimento"=w1030, "column headers"=string[] ["Tiempo EMG(s)", "Amplitud(V)", "Tiempo DPT(s)", "Distancia (cm)", "Potencia optica derecho", "Potencia optica izquierdo"]) -> ()  [unwired: 1 in]
                                }
                              }
                            }
                            frame #2 {
                              # "Si el usuario desea repetir el experimento se vuelve al estado inicio en donde se espera que comience el experimento. De lo contrario se sale del loop y vuelve al menu principal."
                              n546 = Two Button Dialog(message="¿Desea repetir el experimento?", 1:"No" ("F button name (\"Cancel\")"), 2:"Si" ("T button name (\"OK\")")) -> (T button?=w1037:bool)
                              n547 = Not(x=w1037) -> (.not. x?=→"T button?":bool)
                            }
                          }
                        }
                      }
                      n548 = local read "T button?"() -> (w601:bool)
                    }
                  }
                }
                "Array 2" <- w503
              }
            }
          }
          event Timeout {
            n549 = event-data() -> ()  [unwired: 1 in, 3 out]
          }
        }
        "Array 3" <- w31
      }
      "Array 4" <- w22
    }
  }
